vi "Controller.vi"() -> ()   [LabVIEW 2009]
uses:
  <vilib>/regexp/Match Regular Expression.xnode
  <vilib>/gmath/NI_Gmath.lvlib
  <vilib>/Analysis/NI_AALBase.lvlib
panel:
  out "Busy":bool
  in  "Tab Control":enum32{"Controls", "Calibrations", "Errors"}(tab)
  out "Standard Dev.":dbl caption="Std. Dev. (J)" format="%#_4e"
  out "Average":dbl caption="Mean (J)" format="%#_4e"
  in  "Averaging":string(combo)="10 s"
  in  "Tab Control 2":T1(tab)
  in  "Comments":string
  in  "Heads Numbers":i16[](array[numeric])
  in  "Heads":i32(listbox)
  in  "Pulsar Handle":i16
  out "Found?":bool
  out "Pulsar Info":string
  in  "OphirFastX":refnum<k7>(container)
  in  "Refreshing (ms)":i32=10
  in  "Window Time (us)":i32=1000
  in  "Ext. Trigger":bool=TRUE
  in  "Trigger Mode":string(combo)="Falling Edge"
  out "Check Lower Level":bool
  in  "Range (Numeric)":dbl[](array[numeric])
  in  "Max. Power (W)":dbl=12.0
  in  "Max. Energy (J)":dbl=1.2
  in  "Pulse Length":string(combo)
  in  "Wavelength (nm)":string(combo)
  in  "Range":string(combo)
  in  "Mode":string(combo)="Energy"
  in  "Autoscale":bool
  in  "Num 1":i32 min=0 max=9 step=1
  in  "Num 2":i32 min=-1 max=10 step=1
  in  "Num 3":i32 min=-1 max=10 step=1
  in  "Active Channels":T2={"A="=FALSE, "B="=FALSE, "C="=TRUE, "D="=TRUE}
  in  "Delays (s)":dbl[](array[numeric]) min=0.0 max=999.999999999999 format="%#_15f"
  in  "VISA Box":refnum<visa-resource-name>="GPIB0::15::INSTR"
  in  "Manual Mode":bool=TRUE
  in  "Modes":cluster{"A=":u16, "B=":u16, "C=":u16, "D=":u16} {"D=" items=["T0+", "A+", "B+", "C+"]; "C=" items=["T0+", "A+", "B+", "D+"]; "B=" items=["T0+", "A+", "C+", "D+"]; "A=" items=["T0+", "B+", "C+", "D+"]}
  in  "Num 4":i32 min=-1 max=10 step=1
  in  "Num 5":i32 min=-1 max=10 step=1
  in  "Num 6":i32 min=-1 max=10 step=1
  in  "Num 7":i32 min=-1 max=10 step=1
  in  "Num 8":i32 min=-1 max=10 step=1
  in  "Num 9":i32 min=-1 max=10 step=1
  in  "Num 10":i32 min=-1 max=10 step=1
  in  "Num 11":i32 min=-1 max=10 step=1
  in  "Num 12":i32 min=-1 max=10 step=1
  in  "Num 13":i32 min=-1 max=10 step=1
  in  "Num 14":i32 min=-1 max=10 step=1
  in  "Num 15":i32 min=-1 max=10 step=1
  in  "Channel":string(combo)="A"
  in  "Buffer Duration (s)":dbl=2.0
  in  "Add ConfigFile":bool=TRUE
  out "Sub-Buffer (# Points)":i32=5
  out "Error LED":bool
  out "Warning LED":bool
  out "OK LED":bool
  in  "Sub-buffer Sizes":u32[](array[numeric])
  in  "T0 (s)":u32[](array[numeric])
  in  "Simulate Values":bool
  in  "Buffer (units)":string(combo)="Minutes"
  in  "Buffer (size)":u32=5
  in  "Graph style":string(combo)="Chart"
  out "# OK":i32
  out "# Over Range":i32
  out "# Saturated":i32
  out "# Missing Pulses":i32
  out "# Points":i32
  in  "Min. Size (# Points)":i32=5
  in  "Export as .txt":bool
  out "Peak Power (W)":dbl
  out "Peak Energy (J)":dbl
  in  "Step Duration (s)":i32=10
  in  "# Steps":i32=20
  in  "Calibrate":bool
  in  "Rise":string(combo)="Synchronous"
  out "Display":dbl[][](graph)
  out "Measure":dbl caption="Energy (J)" format="%#_4e"
  in  "Slide Style":string(combo)="Absolute"
  in  "Slide (%,W,J)":dbl(slide) caption="Energy (J)" min=0.0 max=1.2 step=0.005 scale=0.0..1.2 scale format="%#_3f"
  in  "Acquire":bool=TRUE
  in  "Clear Graph":bool
  out "Abs Energies":dbl[](array[numeric])
  out "Calib Path":path=path "C:/Documents and Settings/loasis/My Documents/Guillaume/Powermeter/Godzilla Calibrations"
  in  "Titles":string[](array[string])=["Channel A", "Channel B", "Channel C", "Channel D", "Power (W)", "Energy (J)"]
  in  "RmvCalib":bool
  in  "Load list":bool
  in  "AddCalib":bool
  in  "List of calibrations":i32(listbox)=-1
  in  "Calibration":dbl[][](array[numeric])=[[0.000303, 0.000306, 0.000498714, 0.000498713, 0.05, 0.005], [0.000303, 0.000306, 0.000499714, 0.000499713, 0.1, 0.01], [0.000303, 0.000306, 0.000500314, 0.000500413, 0.2, 0.02], [0.000303, 0.000306, 0.000501314, 0.000501413, 0.5, 0.05], [0.000303, 0.000306, 0.000501914, 0.000501813, 1.0, 0.1], [0.000303, 0.000306, 0.000502414, 0.000502213, 2.0, 0.2], [0.000303, 0.000306, 0.000502514, 0.000502513, 3.0, 0.3], [0.000303, 0.000306, 0.000502714, 0.000502613, 4.0, 0.4], [0.000303, 0.000306, 0.000502914, 0.000502813, 5.0, 0.5], [0.000303, 0.000306, 0.000503014, 0.000503013, 6.1, 0.6], [0.000303, 0.000306, 0.000503114, 0.000503113, 7.0, 0.7], [0.000303, 0.000306, 0.000503214, 0.000503213, 8.0, 0.8], [0.000303, 0.000306, 0.000503314, 0.000503313, 9.0, 0.9], [0.000303, 0.000306, 0.000503314, 0.000503413, 9.7, 1.0]]
  out "Indexes":dbl[](array[numeric])
  out "Abs Powers":dbl[](array[numeric])
  in  "Tab Control 3":enum32{"Ophir", "Delay Box", "Saving/Loading"}(tab)
  out "Error Closing USB":errorcluster caption="error out"
  out "Error Getting Data":errorcluster caption="error out"
  out "Error Setting Head":errorcluster caption="error out"
  out "Error Initializing Head":errorcluster caption="error out"
  out "Error Reading Delay Box":errorcluster caption="error out"
  out "Error Writing Delay Box":errorcluster caption="error out"
  out "Error Exporting Text File":errorcluster caption="error out"
  out "Error Loading Dialog":errorcluster caption="error out"
  out "Error Deleting File":errorcluster caption="error out"
  out "Error Writing File":errorcluster caption="error out"
  out "Error Saving Dialog":errorcluster caption="error out"
  in  "Stop":bool
  # "LOASIS/LBNL - Power/Energy-meter Controller - Guillaume Plateau - Version 2.14 - May 2nd, 2010"
  # "(s)"
  # "(ms)"
  # "(us)"
  # "(ns)"
  # "(ps)"
  # "."
  # "Ophir Messages:"
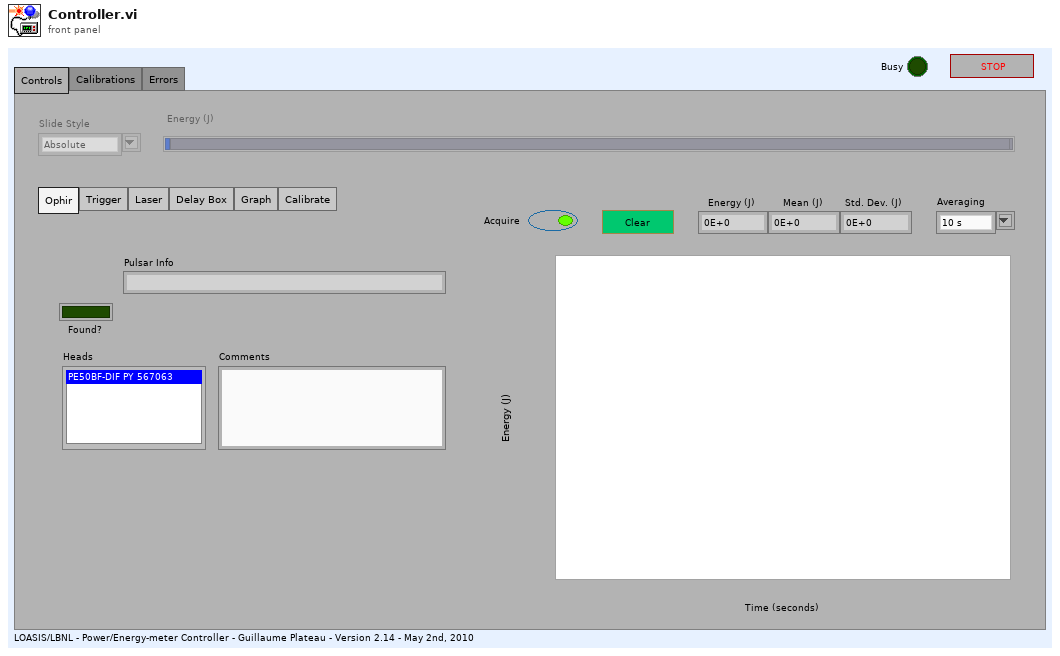
[diagram p1: front panel]
types:
  T1 = enum32{"Ophir", "Trigger", "Laser", "Delay Box", "Graph", "Calibrate"}
  T2 = cluster{"A=":bool, "B=":bool, "C=":bool, "D=":bool}
  T3 = cluster{"Ext. Trigger":bool, "Autoscale":bool, "Check Lower Level":bool, "VISA Box":refnum<visa-resource-name>, "Manual Mode":bool, "Delays (s)":dbl[], "Modes":cluster{"A=":u16, "B=":u16, "C=":u16, "D=":u16}, "Active Channels":cluster{"A=":bool, "B=":bool, "C=":bool, "D=":bool}, "Graph style":string, "Buffer (size)":u32, "Buffer (units)":string, "Min. Size (# Points)":i32, "Simulate Values":bool, "Calib Path":path, "Slide Style":string, "Max. Power (W)":dbl, "Max. Energy (J)":dbl, "Slide (%,W,J)":dbl, "Acquire":bool}
  T4 = cluster{"Ext. Trigger":bool, "Autoscale":bool, "Check Lower Level":bool, "VISA Box":refnum<visa-resource-name>, "Manual Mode":bool, "Delays (s)":dbl[], "Modes":cluster{"A=":u16, "B=":u16, "C=":u16, "D=":u16}, "Active Channels":cluster{"A=":bool, "B=":bool, "C=":bool, "D=":bool}, "Graph style":string, "Buffer (size)":u32, "Buffer (units)":string, "Min. Size (# Points)":i32, "Simulate Values":bool, "Calib Path":path, "Slide Style":string, "Max. Power (W)":dbl, "Max. Energy (J)":dbl, "Slide (%,W,J)":dbl, "Acquire":bool}[]
  T5 = cluster{"Graph (main buffer)":dbl[], "Times (main buffer)":u32[], "Graph (sub-buffer)":dbl[], "Times (sub-buffer)":u32[]}
  T6 = cluster{"Graph (main buffer)":dbl[], "Times (main buffer)":u32[], "Graph (sub-buffer)":dbl[], "Times (sub-buffer)":u32[]}[]
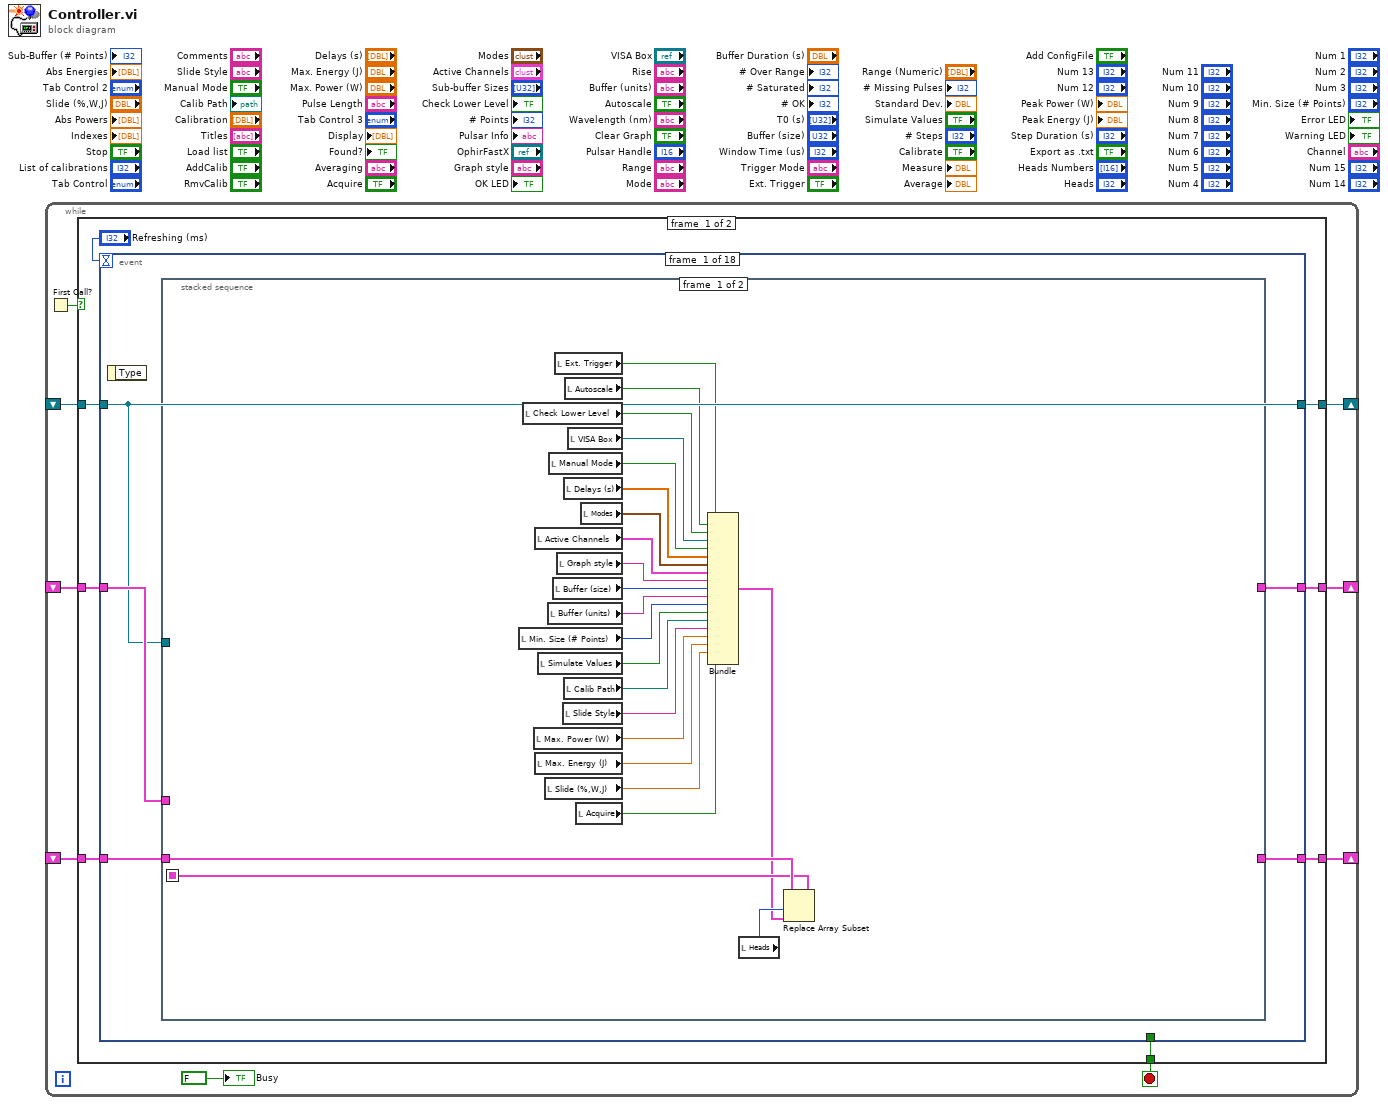
[diagram p0: block diagram]
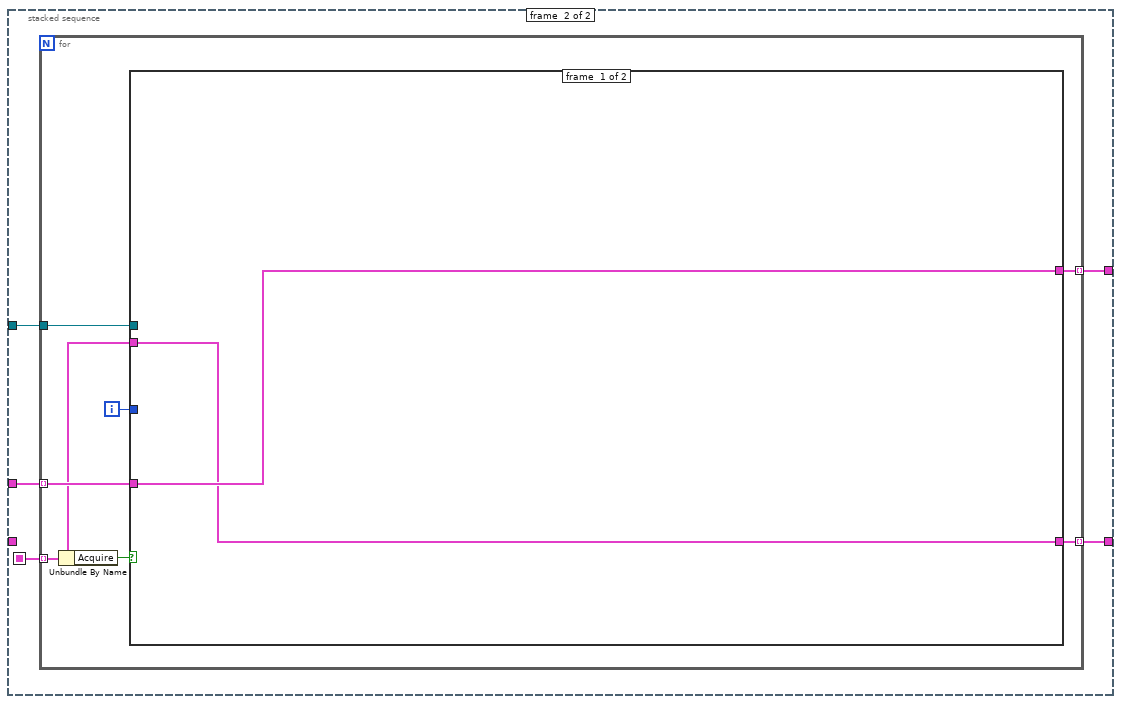
[diagram p2: hidden frame]
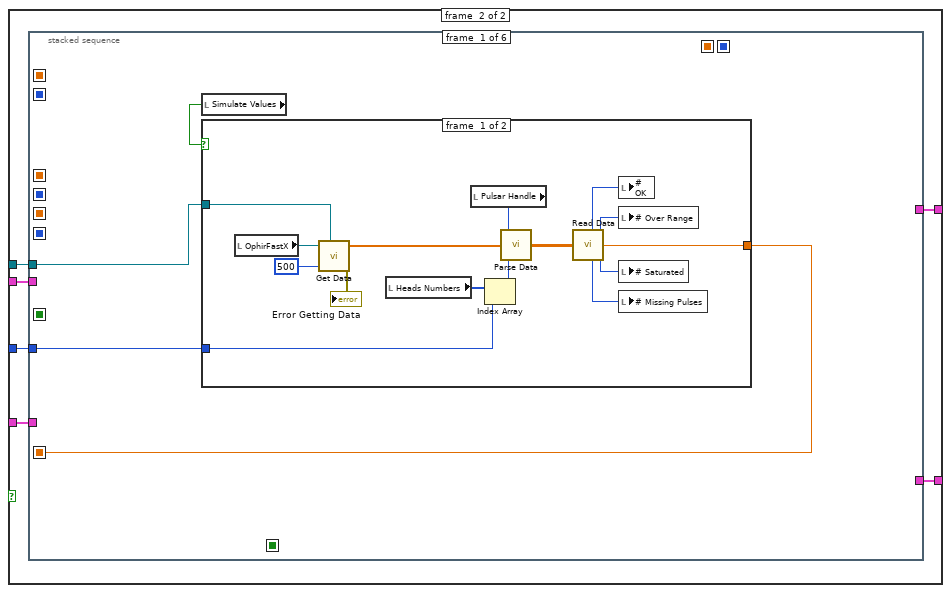
[diagram p3: hidden frame]
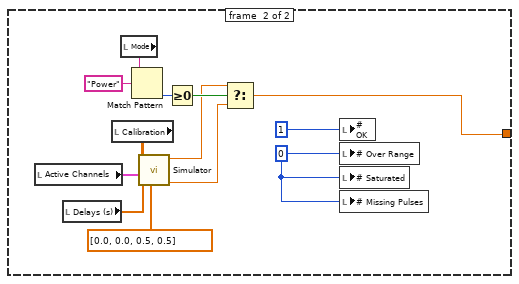
[diagram p4: hidden frame]
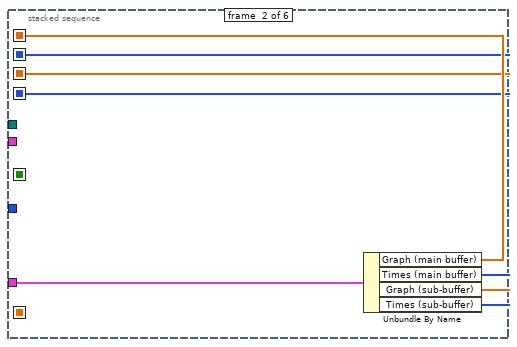
[diagram p5: hidden frame]
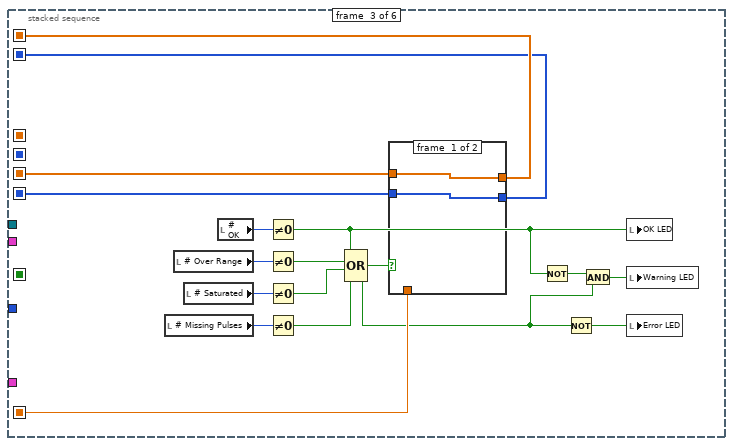
[diagram p6: hidden frame]
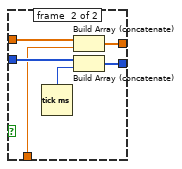
[diagram p7: hidden frame]
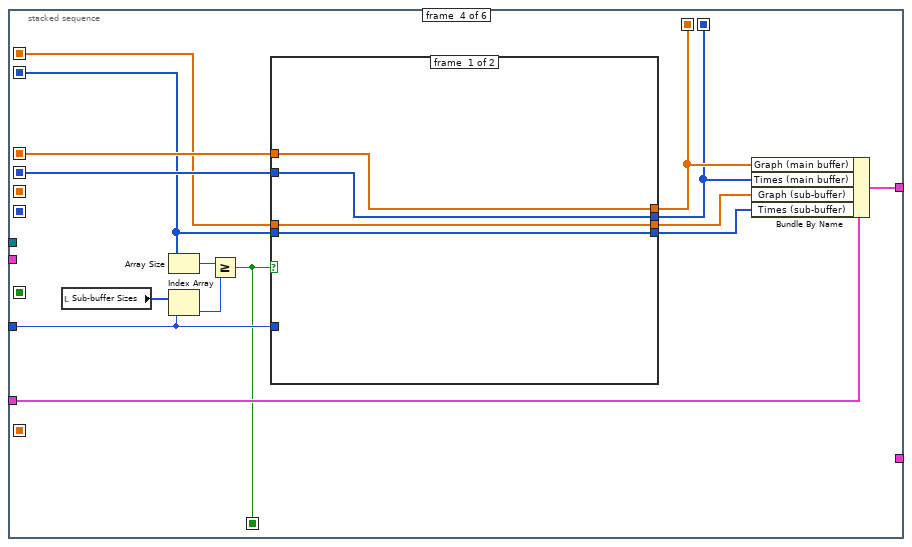
[diagram p8: hidden frame]
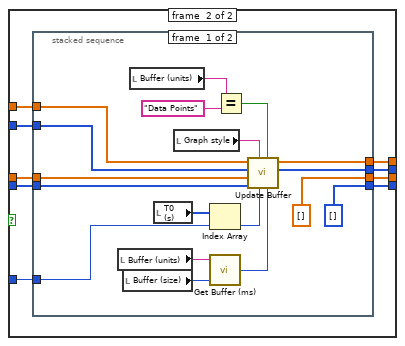
[diagram p9: hidden frame]
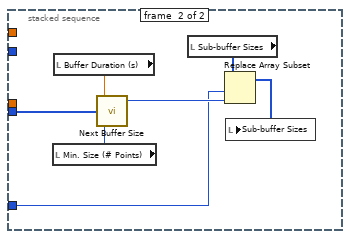
[diagram p10: hidden frame]
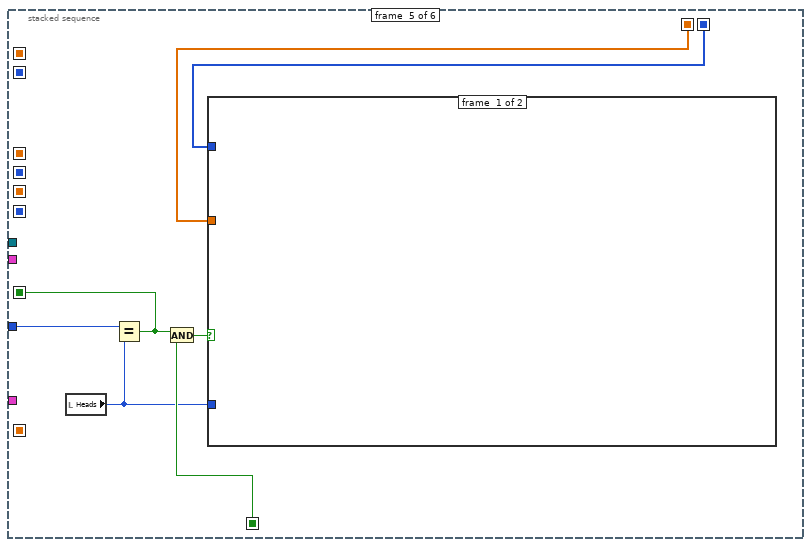
[diagram p11: hidden frame]
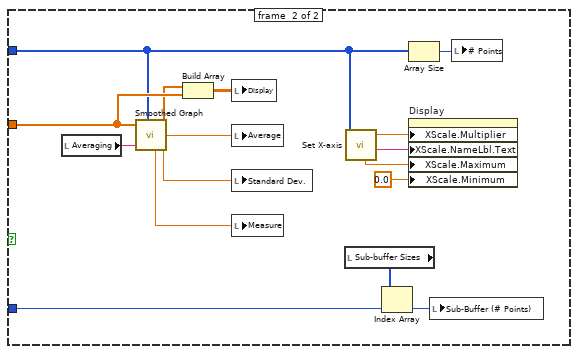
[diagram p12: hidden frame]
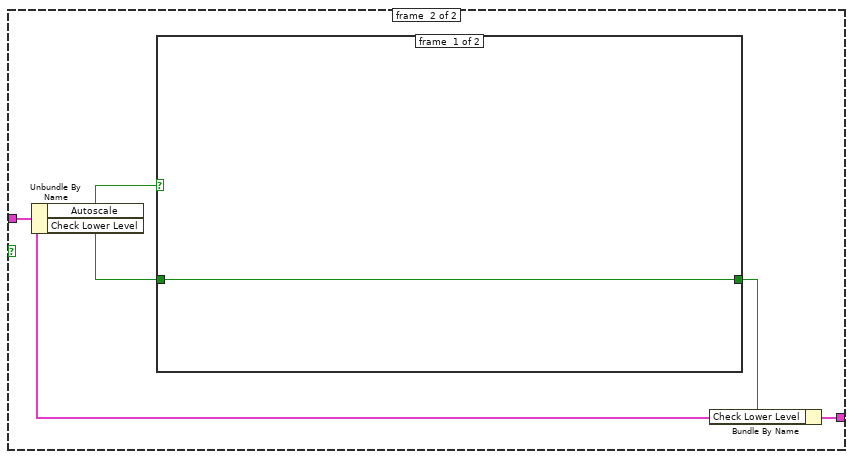
[diagram p14: hidden frame]
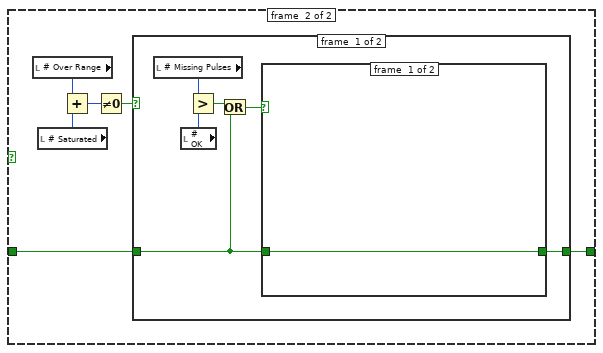
[diagram p15: hidden frame]
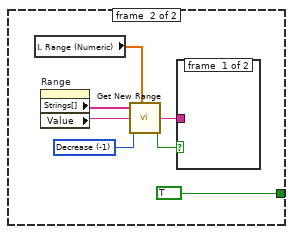
[diagram p16: hidden frame]
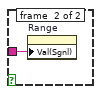
[diagram p17: hidden frame]
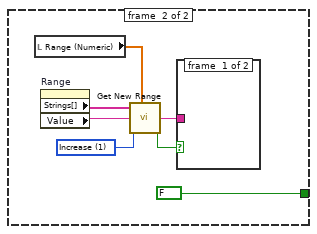
[diagram p18: hidden frame]
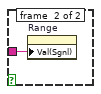
[diagram p19: hidden frame]
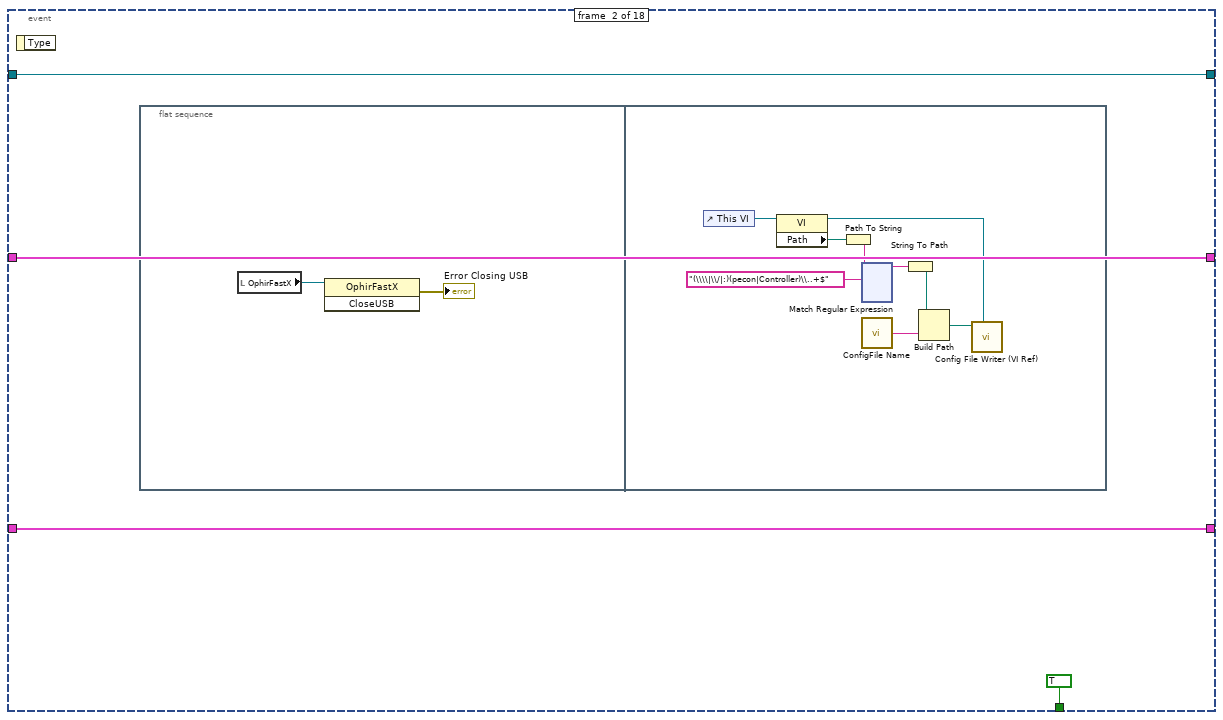
[diagram p20: hidden frame]
diagram:
  n1 = while {
    shift-right: [w7] -> _
    shift-left: _ -> [w6]
    shift-right: [w2] -> _
    shift-left: _ -> [w4]
    shift-right: [w1] -> _
    shift-left: _ -> [w3]
    stop <- w8 stop-if-true
    n2 = First Call?() -> (First Call?: T/F=w5:bool)
    n3 = case shown="False" w5 {
      tunnel: [w17 FALSE ("stop")] -> w8
      tunnel: [w11 w2302] -> w7
      tunnel: w6 -> [w12 _]
      tunnel: w3 -> [w13 w2299]
      tunnel: w4 -> [w15 _]
      tunnel: [w14 w2301] -> w2
      tunnel: [w10 w2300] -> w1
      frame #0 {
        n4 = event shown="[1] \"Stop\": Mouse Up" {
          selector: _ -> [_ _ _ _ _ _ _ _ _ _ _ _ _ _ _ _ _ _]
          dyn-events: _ -> [_ _ _ _ _ _ _ _ _ _ _ _ _ _ _ _ _ _]
          timeout: "Refreshing (ms)" -> [_ _ _ _ _ _ _ _ _ _ _ _ _ _ _ _ _ _]
          tunnel: [_ TRUE ("stop") _ _ _ _ _ _ _ _ _ _ _ _ _ _ _ _] -> w17
          tunnel: w15 -> [w21 w245 w366 w410 w424 w1004 w1060 w1112 w1149 w1291 w1351 w1403 w1791 w1818 w1847 w1884 w2220 w2286]
          tunnel: [w19 w245 w366 w409 w424 w1004 w1060 w1112 w1149 w1291 w1351 w1403 w1791 w1818 w1847 w1884 w2220 w2286] -> w14
          tunnel: w13 -> [w22 w243 w367 w407 w422 w1002 w1058 w1110 w1147 w1289 w1349 w1401 w1789 w1816 w1845 w1883 w2218 w2284]
          tunnel: w12 -> [w20 w244 w368 w408 w423 w1003 w1059 w1111 w1148 w1290 w1350 w1402 w1790 w1817 w1846 w1885 w2219 w2285]
          tunnel: [w20 w244 w368 w408 w423 w1003 w1059 w1111 w1148 w1290 w1350 w1402 w1790 w1817 w1846 w1885 w2219 w2285] -> w11
          tunnel: [w18 w243 w367 w407 w422 w1002 w1058 w1110 w1147 w1289 w1349 w1401 w1789 w1816 w1845 w1883 w2218 w2284] -> w10
          event #0 {
            n5 = event-data() -> ()  [unwired: 1 in, 1 out]
            n6 = stacked-sequence {
              seq-local: [w43 _] -> [_ w47]
              tunnel: w22 -> [w44 _]
              tunnel: [_ w50] -> w18
              tunnel: w20 -> [_ w49]
              tunnel: w21 -> [_ w48]
              tunnel: [_ w46] -> w19
              frame #0 {
                n7 = local read "Min. Size (# Points)"() -> (w24:i32)
                n8 = local read "Check Lower Level"() -> (w30:bool)
                n9 = local read "Max. Power (W)"() -> (w28:dbl)
                n10 = local read "Active Channels"() -> (w29:T2)
                n11 = local read "Max. Energy (J)"() -> (w27:dbl)
                n12 = local read "Simulate Values"() -> (w34:bool)
                n13 = local read "Slide (%,W,J)"() -> (w26:dbl)
                n14 = local read "Buffer (units)"() -> (w33:string)
                n15 = local read "Manual Mode"() -> (w39:bool)
                n16 = local read "Buffer (size)"() -> (w32:u32)
                n17 = local read "Ext. Trigger"() -> (w42:bool)
                n18 = local read "Graph style"() -> (w25:string)
                n19 = local read "Slide Style"() -> (w36:string)
                n20 = local read "Delays (s)"() -> (w38:dbl[])
                n21 = local read "Calib Path"() -> (w35:path)
                n22 = local read "Autoscale"() -> (w41:bool)
                n23 = local read "VISA Box"() -> (w40:refnum<visa-resource-name>)
                n24 = local read "Acquire"() -> (w37:bool)
                n25 = local read "Modes"() -> (w31:cluster{"A=":u16, "B=":u16, "C=":u16, "D=":u16})
                n26 = Bundle("Ext. Trigger"=w42, "Autoscale"=w41, "Check Lower Level"=w30, "VISA Box"=w40, "Manual Mode"=w39, "Delays (s)"=w38, "Modes"=w31, "Active Channels"=w29, "Graph style"=w25, "Buffer (size)"=w32, "Buffer (units)"=w33, "Min. Size (# Points)"=w24, "Simulate Values"=w34, "Calib Path"=w35, "Slide Style"=w36, "Max. Power (W)"=w28, "Max. Energy (J)"=w27, "Slide (%,W,J)"=w26, "Acquire"=w37) -> (w23:T3)  [unwired: 1 in]
                n27 = local read "Heads"() -> (w45:i32)
                n28 = Replace Array Subset(array=w44, new element=w23, index=w45) -> (w43:T4)
              }
              frame #1 {
                n29 = for {
                  tunnel: w49 -> [w57]
                  tunnel: w48 -> [w56] mode=indexing
                  tunnel: [w55] -> w46 mode=indexing
                  tunnel: w47 -> [w52] mode=indexing
                  tunnel: [w51] -> w50 mode=indexing
                  i -> [w54]
                  n30 = Unbundle By Name(w52) -> ("Acquire"=w53:bool)
                  n31 = case shown="True" w53 {
                    tunnel: w57 -> [_ w65]
                    tunnel: w56 -> [w59 w64]
                    tunnel: [w59 w63] -> w55
                    tunnel: w54 -> [_ w62]
                    tunnel: w52 -> [w58 w61]
                    tunnel: [w58 w60] -> w51
                    frame #0 {
                    }
                    frame #1 {
                      n32 = stacked-sequence {
                        seq-local: [_ w101 _ _ _ _] -> [_ _ _ w138 _ _]
                        seq-local: [_ w100 _ _ _ _] -> [_ _ _ w137 _ _]
                        seq-local: [_ w99 _ _ _ _] -> [_ _ w112 _ _ _]
                        seq-local: [_ w98 _ _ _ _] -> [_ _ w111 _ _ _]
                        seq-local: [_ _ w109 _ _ _] -> [_ _ _ w135 _ _]
                        seq-local: [_ _ w108 _ _ _] -> [_ _ _ w136 _ _]
                        seq-local: [_ _ _ w129 _ _] -> [_ _ _ _ w187 _]
                        seq-local: [_ _ _ w130 _ _] -> [_ _ _ _ w186 _]
                        seq-local: [_ _ _ w128 _ _] -> [_ _ _ _ w184 _]
                        seq-local: [w66 _ _ _ _ _] -> [_ _ w110 _ _ _]
                        seq-local: [_ _ _ _ w182 _] -> [_ _ _ _ _ w205]
                        tunnel: w65 -> [w69 _ _ _ _ _]
                        tunnel: w64 -> [_ w102 _ w134 _ _]
                        tunnel: w62 -> [w68 _ _ w139 w185 _]
                        tunnel: [_ _ _ w131 _ _] -> w63
                        tunnel: w61 -> [_ _ _ _ _ w206]
                        tunnel: [_ _ _ _ _ w204] -> w60
                        frame #0 {
                          n33 = local read "Simulate Values"() -> (w67:bool)
                          n34 = case shown="False" w67 {
                            tunnel: [w75 w86] -> w66
                            tunnel: w69 -> [w71 _]
                            tunnel: w68 -> [w70 _]
                            frame #0 {
                              n35 = local read "OphirFastX"() -> (w72:refnum<k7>)
                              n36 = call "Get Data.vi"("OphirFastX"=w72, "Notifier"=w71, "Timeout (ms)"=500 ("timeout in ms (-1)")) -> ("Data"=w81:dbl[], "Error"=→"Error Getting Data":errorcluster)  [unwired: 5 in]
                              n37 = local read "Heads Numbers"() -> (w74:i16[])
                              n38 = local read "Pulsar Handle"() -> (w82:i16)
                              n39 = Index Array(array=w74, index=w70) -> (element=w73:i16)
                              n40 = call "Parse Data.vi"("Head Channel"=w73, "Raw Data"=w81, "Pulsar Handle"=w82) -> ("Selected data"=w80:dbl[][])  [unwired: 2 in]
                              n41 = call "Read Data.vi"("Selected data"=w80) -> ("# OK"=w77:i32, "# Over Range"=w79:i32, "Data Point"=w75:dbl, "# Missing Pulses"=w76:i32, "# Saturated"=w78:i32)  [unwired: 4 in]
                              n42 = local write "# OK"(w77) -> ()
                              n43 = local write "# Over Range"(w79) -> ()
                              n44 = local write "# Saturated"(w78) -> ()
                              n45 = local write "# Missing Pulses"(w76) -> ()
                            }
                            frame #1 {
                              w87 = 0 ("# Over Range")
                              n46 = local read "Active Channels"() -> (w85:T2)
                              n47 = local read "Delays (s)"() -> (w96:dbl[])
                              n48 = local read "Calibration"() -> (w97:dbl[][])
                              n49 = local read "Mode"() -> (w94:string)
                              n50 = Match Pattern(string=w94, regular expression="Power") -> (offset past match=w92:i32)  [unwired: 1 in, 3 out]
                              n51 = call "Simulator.vi"("Proportions"=dbl[] [0.0, 0.0, 0.5, 0.5], "Delays (s)"=w96, "Active Channels"=w85, "Calibration"=w97) -> ("Output Energy (J)"=w89:dbl, "Output Power (W)"=w90:dbl)  [unwired: 6 in]
                              n52 = Greater Or Equal To 0?(x=w92) -> (x >= 0?=w91:bool)
                              n53 = Select(t=w90, s=w91, f=w89) -> (s? t:f=w86:dbl)
                              n54 = local write "# OK"(1 ("# OK")) -> ()
                              n55 = local write "# Over Range"(w87) -> ()
                              n56 = local write "# Saturated"(w87) -> ()
                              n57 = local write "# Missing Pulses"(w87) -> ()
                            }
                          }
                        }
                        frame #1 {
                          n58 = Unbundle By Name(w102) -> ("Graph (main buffer)"=w101:dbl[], "Times (main buffer)"=w100:u32[], "Graph (sub-buffer)"=w99:dbl[], "Times (sub-buffer)"=w98:u32[])
                        }
                        frame #2 {
                          n59 = local read "# Missing Pulses"() -> (w116:i32)
                          n60 = local read "# Over Range"() -> (w118:i32)
                          n61 = local read "# Saturated"() -> (w117:i32)
                          n62 = local read "# OK"() -> (w119:i32)
                          n63 = Not Equal To 0?(x=w119) -> (x != 0?=w106:bool)
                          n64 = Not Equal To 0?(x=w118) -> (x != 0?=w114:bool)
                          n65 = Not Equal To 0?(x=w117) -> (x != 0?=w113:bool)
                          n66 = Not Equal To 0?(x=w116) -> (x != 0?=w115:bool)
                          n67 = Compound Arithmetic op=OR(w106, w114, w113, w115) -> (w104:bool)
                          n68 = case shown="True" w104 {
                            tunnel: w112 -> [w121 w126]
                            tunnel: w111 -> [w120 w125]
                            tunnel: w110 -> [_ w124]
                            tunnel: [w121 w123] -> w109
                            tunnel: [w120 w122] -> w108
                            frame #0 {
                            }
                            frame #1 {
                              n69 = Tick Count (ms)() -> (millisecond timer value=w127:u32)
                              n70 = Build Array (concatenate)(w126, w124) -> (w123:dbl[])
                              n71 = Build Array (concatenate)(w125, w127) -> (w122:u32[])
                            }
                          }
                          n72 = Not(x=w106) -> (.not. x?=w105:bool)
                          n73 = Not(x=w104) -> (.not. x?=w107:bool)
                          n74 = And(x=w105, y=w104) -> (x .and. y?=w103:bool)
                          n75 = local write "OK LED"(w106) -> ()
                          n76 = local write "Warning LED"(w103) -> ()
                          n77 = local write "Error LED"(w107) -> ()
                        }
                        frame #3 {
                          n78 = local read "Sub-buffer Sizes"() -> (w141:u32[])
                          n79 = Array Size(array=w136) -> (size(s)=w142:i32)
                          n80 = Index Array(array=w141, index=w139) -> (element=w140:u32)
                          n81 = Greater Or Equal?(x=w142, y=w140) -> (x >= y?=w128:bool)
                          n82 = case shown="True" w128 {
                            tunnel: w139 -> [_ w155]
                            tunnel: w138 -> [w144 w150]
                            tunnel: w137 -> [w143 w149]
                            tunnel: w136 -> [w145 w154]
                            tunnel: w135 -> [w146 w153]
                            tunnel: [w144 w152] -> w130
                            tunnel: [w143 w151] -> w129
                            tunnel: [w146 w148] -> w133
                            tunnel: [w145 w147] -> w132
                            frame #0 {
                            }
                            frame #1 {
                              n83 = stacked-sequence {
                                tunnel: w155 -> [w165 w177]
                                tunnel: w154 -> [w163 w178]
                                tunnel: w153 -> [w162 _]
                                tunnel: [w161 _] -> w152
                                tunnel: [w160 _] -> w151
                                tunnel: w150 -> [w159 _]
                                tunnel: w149 -> [w158 _]
                                tunnel: [dbl[] [] ("Graph (out)") _] -> w148
                                tunnel: [u32[] [] ("Times (out)") _] -> w147
                                frame #0 {
                                n84 = local read "Buffer (units)"() -> (w173:string)
                                n85 = local read "Buffer (size)"() -> (w172:u32)
                                n86 = local read "Buffer (units)"() -> (w169:string)
                                n87 = local read "T0 (s)"() -> (w166:u32[])
                                n88 = local read "Graph style"() -> (w170:string)
                                n89 = Index Array(array=w166, index=w165) -> (element=w164:u32)
                                n90 = call "Get Buffer (ms).vi"("Buffer (size)"=w172, "Buffer (units)"=w173) -> ("Buffer (ms)"=w171:u32)  [unwired: 3 in]
                                n91 = Equal?(x=w169, y="Data Points") -> (x = y?=w167:bool)
                                n92 = call "Update Buffer.vi"("Buffer (ms)"=w171, "Data Points mode"=w167, "T0 (s)"=w164, "Graph style"=w170, "Times to add"=w163, "Values to add"=w162, "Times (in)"=w158, "Graph (in)"=w159) -> ("Times (out)"=w160:u32[], "Graph (out)"=w161:dbl[])  [unwired: 2 in]
                                }
                                frame #1 {
                                n93 = local read "Min. Size (# Points)"() -> (w176:i32)
                                n94 = local read "Buffer Duration (s)"() -> (w174:dbl)
                                n95 = call "Next Buffer Size.vi"("Min Size"=w176, "Times"=w178, "Buffer Duration (s)"=w174) -> ("Next buffer size"=w179:i32)  [unwired: 1 in, 1 out]
                                n96 = local read "Sub-buffer Sizes"() -> (w180:u32[])
                                n97 = Replace Array Subset(array=w180, new element=w179, index=w177) -> (w175:u32[])
                                n98 = local write "Sub-buffer Sizes"(w175) -> ()
                                }
                              }
                            }
                          }
                          n99 = Bundle By Name(cluster=w134, "Graph (main buffer)"=w130, "Times (main buffer)"=w129, "Graph (sub-buffer)"=w133, "Times (sub-buffer)"=w132) -> (w131:T5)
                        }
                        frame #4 {
                          n100 = local read "Heads"() -> (w181:i32)
                          n101 = Equal?(x=w185, y=w181) -> (x = y?=w182:bool)
                          n102 = And(x=w182, y=w184) -> (x .and. y?=w183:bool)
                          n103 = case shown="True" w183 {
                            tunnel: w186 -> [_ w201]
                            tunnel: w187 -> [_ w195]
                            tunnel: w181 -> [_ w188]
                            frame #0 {
                            }
                            frame #1 {
                              n104 = local read "Averaging"() -> (w202:string)
                              n105 = call "Smoothed Graph.vi"("Raw Graph"=w201, "Times"=w195, "Averaging"=w202) -> ("Avg Graph"=w200:dbl[], "Mean"=w198:dbl, "Last Value"=w197:dbl, "Std. Dev."=w196:dbl)  [unwired: 3 in]
                              n106 = Build Array(w200, w201) -> (w199:dbl[][])
                              n107 = local write "Display"(w199) -> ()
                              n108 = local write "Average"(w198) -> ()
                              n109 = local write "Standard Dev."(w196) -> ()
                              n110 = local write "Measure"(w197) -> ()
                              n111 = local read "Sub-buffer Sizes"() -> (w189:u32[])
                              n112 = call "Set X-axis.vi"("Times"=w195) -> ("X-label"=w193:string, "Multiplier"=w203:dbl, "X-Scale Maximum"=w192:dbl)  [unwired: 8 in]
                              n113 = Index Array(array=w189, index=w188) -> (element=w190:u32)
                              n114 = Array Size(array=w195) -> (size(s)=w194:i32)
                              n115 = property on="Display" class="WFGraph (strict)"("XScale.Multiplier"=w203, "XScale.NameLbl.Text"=w193, "XScale.Maximum"=w192, "XScale.Minimum"=0.0 ("X Scale.Range:Minimum")) -> ()  [unwired: 2 in, 2 out]
                              n116 = local write "Sub-Buffer (# Points)"(w190) -> ()
                              n117 = local write "# Points"(w194) -> ()
                            }
                          }
                        }
                        frame #5 {
                          n118 = case shown="True" w205 {
                            tunnel: w206 -> [w207 w208]
                            tunnel: [w207 w209] -> w204
                            frame #0 {
                            }
                            frame #1 {
                              n119 = Unbundle By Name(w208) -> ("Autoscale"=w212:bool, "Check Lower Level"=w211:bool)
                              n120 = case shown="True" w212 {
                                tunnel: w211 -> [w213 w215]
                                tunnel: [w213 w214] -> w210
                                frame #0 {
                                }
                                frame #1 {
                                n121 = local read "# Over Range"() -> (w219:i32)
                                n122 = local read "# Saturated"() -> (w218:i32)
                                n123 = Add(x=w219, y=w218) -> (x+y=w217:i32)
                                n124 = Not Equal To 0?(x=w217) -> (x != 0?=w216:bool)
                                n125 = case shown="False" w216 {
                                tunnel: w215 -> [w220 _]
                                tunnel: [w221 FALSE ("Check Lower Level")] -> w214
                                frame #0 {
                                n126 = local read "# Missing Pulses"() -> (w225:i32)
                                n127 = local read "# OK"() -> (w224:i32)
                                n128 = Greater?(x=w225, y=w224) -> (0:w223:bool)
                                n129 = Or(x=w223, y=w220) -> (x .or. y?=w222:bool)
                                n130 = case shown="True" w222 {
                                tunnel: [w226 TRUE ("Check Lower Level")] -> w221
                                tunnel: w220 -> [w226 _]
                                frame #0 {
                                }
                                frame #1 {
                                w231 = -1 items=["Decrease"=-1, "Increase"=1, "None"=0] ("Action")
                                n131 = local read "Range (Numeric)"() -> (w227:dbl[])
                                n132 = property on="Range" class="CmbBox"() -> ("Strings[]"=w233:string[], "Value"=w232:string)  [unwired: 2 in, 2 out]
                                n133 = call "Get New Range.vi"("Ranges"=w233, "Range (numeric)"=w227, "Range (char)"=w232, "Action"=w231) -> ("New Range"=w230:string, "New?"=w228:bool)  [unwired: 4 in]
                                n134 = case shown="True" w228 {
                                tunnel: w230 -> [_ w234]
                                frame #0 {
                                }
                                frame #1 {
                                n135 = property on="Range" class="CmbBox"("Val(Sgnl)"=w234) -> ()  [unwired: 2 in, 2 out]
                                }
                                }
                                }
                                }
                                }
                                frame #1 {
                                w239 = 1 items=["Decrease"=-1, "Increase"=1, "None"=0] ("Action")
                                n136 = local read "Range (Numeric)"() -> (w235:dbl[])
                                n137 = property on="Range" class="CmbBox"() -> ("Strings[]"=w241:string[], "Value"=w240:string)  [unwired: 2 in, 2 out]
                                n138 = call "Get New Range.vi"("Ranges"=w241, "Range (numeric)"=w235, "Range (char)"=w240, "Action"=w239) -> ("New Range"=w238:string, "New?"=w236:bool)  [unwired: 4 in]
                                n139 = case shown="True" w236 {
                                tunnel: w238 -> [_ w242]
                                frame #0 {
                                }
                                frame #1 {
                                n140 = property on="Range" class="CmbBox"("Val(Sgnl)"=w242) -> ()  [unwired: 2 in, 2 out]
                                }
                                }
                                }
                                }
                                }
                              }
                              n141 = Bundle By Name(cluster=w208, "Check Lower Level"=w210) -> (w209:T3)
                            }
                          }
                        }
                      }
                    }
                  }
                }
              }
            }
          }
          event #1 {
            n142 = event-data() -> ()  [unwired: 1 in, 1 out]
            n143 = flat-sequence {
              frame #0 {
                n144 = local read "OphirFastX"() -> (w248:refnum<k7>)
                n145 = invoke class="OphirFastX" method="CloseUSB"(reference=w248) -> (error out=→"Error Closing USB":errorcluster)  [unwired: 2 in, 2 out]
              }
              frame #1 {
                n146 = control-ref of="This VI"() -> (w257:refnum<vi>)
                n147 = property class="VI"(reference=w257) -> (reference out=w256:refnum<vi>, "Path"=w253:path)  [unwired: 1 in, 1 out]
                n148 = Path To String(path=w253) -> (string=w252:string)
                n149 = xnode "Match Regular Expression"("input string"=w252, "regular expression"="(\\\\|\\/|:)(pecon|Controller)\\..+$") -> ("before match"=w251:string)  [unwired: 4 in, 4 out]
                n150 = call "ConfigFile Name.vi"() -> ("ConfigFile Name"=w255:string)  [unwired: 5 in]
                n151 = String To Path(string=w251) -> (path=w250:path)
                n152 = Build Path(base path=w250, name or relative path=w255) -> (appended path=w249:path)
                n153 = call "Config File Writer (VI Ref).vi"("This VI"=w256, "Config File Path"=w249) -> ()  [unwired: 9 in, 1 out]
              }
            }
          }
          event #2 {
            n154 = event-data() -> ()  [unwired: 1 in, 1 out]
            n155 = flat-sequence {
              tunnel: w366 -> [w395]
              tunnel: [w373] -> w365
              tunnel: w365 -> [w396]
              frame #0 {
                w382 = "\t"
                n156 = local read "Heads"() -> (w393:i32)
                n157 = local read "Averaging"() -> (w369:string)
                n158 = Index Array(array=w395, index=w393) -> (element=w392:T5)
                n159 = property on="Display" class="WFGraph (strict)"() -> ("YScale.NameLbl.Text"=w371:string)  [unwired: 2 in, 2 out]
                n160 = Unbundle By Name(w392) -> ("Graph (main buffer)"=w380:dbl[], "Times (main buffer)"=w379:u32[])
                n161 = Concatenate Strings(w369, " Averaged " ("string"), w371) -> (w372:string)
                n162 = Array Size(array=w379) -> (size(s)=w391:i32)
                n163 = call "Set X-axis.vi"("Times"=w379) -> ("X-label"=w384:string, "Multiplier"=w390:dbl)  [unwired: 8 in, 1 out]
                n164 = Concatenate Strings(w384, w382, w371, w382, w372, "\r\n") -> (w377:string)
                n165 = local read "Averaging"() -> (w381:string)
                n166 = call <vilib>:"Ramp Pattern.vi"("samples"=w391) -> ("Ramp Pattern"=w389:dbl[])  [unwired: 9 in, 1 out]
                n167 = local write "Busy"(TRUE ("Busy")) -> ()
                n168 = Multiply(x=w390, y=w389) -> (x*y=w388:dbl[])
                n169 = call "Smoothed Graph.vi"("Raw Graph"=w380, "Times"=w379, "Averaging"=w381) -> ("Avg Graph"=w378:dbl[])  [unwired: 3 in, 3 out]
                n170 = Build Array(w388, w380, w378) -> (w387:dbl[][])
                n171 = Transpose 2D Array(2D array=w387) -> (transposed array=w385:dbl[][])
                n172 = Array To Spreadsheet String(array=w385, 3:"%3.12e" ("format string")) -> (spreadsheet string=w376:string)  [unwired: 1 in]
                n173 = Concatenate Strings(w377, w376) -> (w375:string)
                n174 = Write to Text File(text=w375) -> (refnum out=w373:refnum<file>, error out=→"Error Exporting Text File":errorcluster)  [unwired: 3 in, 1 out]
              }
              frame #1 {
                n175 = Not A Number/Path/Refnum?(number/path/refnum=w396) -> (NaN/Path/Refnum?=w400:bool)
                n176 = Not(x=w400) -> (.not. x?=w399:bool)
                n177 = local read "Add ConfigFile"() -> (w398:bool)
                n178 = Or(x=w398, y=w399) -> (x .or. y?=w397:bool)
                n179 = case shown="True" w397 {
                  tunnel: w396 -> [_ w401]
                  frame #0 {
                  }
                  frame #1 {
                    n180 = Close File(refnum=w401) -> (path=w403:path)  [unwired: 1 in, 1 out]
                    n181 = call "ConfigFile Name.vi"() -> ("ConfigFile Name"=w406:string)  [unwired: 5 in]
                    n182 = Strip Path(path=w403) -> (stripped path=w402:path)  [unwired: 1 out]
                    n183 = Build Path(base path=w402, name or relative path=w406) -> (appended path=w405:path)
                    n184 = control-ref of="This VI"() -> (w404:refnum<vi>)
                    n185 = call "Config File Writer (VI Ref).vi"("This VI"=w404, "Config File Path"=w405) -> ()  [unwired: 9 in, 1 out]
                  }
                }
              }
            }
          }
          event #3 {
            w420 = u32[] []  # Times (sub-buffer)
            w419 = dbl[] []  # Graph (sub-buffer)
            w418 = u32[] []  # Times (main buffer)
            w417 = dbl[] []  # Graph (main buffer)
            n186 = event-data() -> ()  [unwired: 1 in, 1 out]
            n187 = local write "Busy"(TRUE ("Busy")) -> ()
            n188 = Bundle("Graph (main buffer)"=w417, "Times (main buffer)"=w418, "Graph (sub-buffer)"=w419, "Times (sub-buffer)"=w420) -> (w416:T5)  [unwired: 1 in]
            n189 = local read "Heads"() -> (w421:i32)
            n190 = Replace Array Subset(array=w410, new element=w416, index=w421) -> (w409:T6)
            n191 = Tick Count (ms)() -> (millisecond timer value=w412:u32)
            n192 = local read "Heads"() -> (w414:i32)
            n193 = local read "T0 (s)"() -> (w413:u32[])
            n194 = Replace Array Subset(array=w413, new element=w412, index=w414) -> (w411:u32[])
            n195 = local write "T0 (s)"(w411) -> ()
          }
          event #4 {
            n196 = event-data() -> ()  [unwired: 1 in, 1 out]
            n197 = stacked-sequence {
              tunnel: w422 -> [w445 _ _ _ _ _ _ _ _]
              frame #0 {
                n198 = local write "Busy"(TRUE ("Busy")) -> ()
                n199 = local read "Heads"() -> (w447:i32)
                n200 = Index Array(array=w445, index=w447) -> (element=w425:T3)
                n201 = Unbundle(w425) -> ("Ext. Trigger"=w444:bool, "Autoscale"=w443:bool, "Check Lower Level"=w432:bool, "VISA Box"=w442:refnum<visa-resource-name>, "Manual Mode"=w441:bool, "Delays (s)"=w440:dbl[], "Modes"=w433:cluster{"A=":u16, "B=":u16, "C=":u16, "D=":u16}, "Active Channels"=w431:T2, "Graph style"=w427:string, "Buffer (size)"=w434:u32, "Buffer (units)"=w435:string, "Min. Size (# Points)"=w426:i32, "Simulate Values"=w436:bool, "Calib Path"=w437:path, "Slide Style"=w438:string, "Max. Power (W)"=w430:dbl, "Max. Energy (J)"=w429:dbl, "Slide (%,W,J)"=w428:dbl, "Acquire"=w439:bool)
                n202 = local write "Ext. Trigger"(w444) -> ()
                n203 = local write "Autoscale"(w443) -> ()
                n204 = local write "Check Lower Level"(w432) -> ()
                n205 = local write "VISA Box"(w442) -> ()
                n206 = local write "Manual Mode"(w441) -> ()
                n207 = local write "Delays (s)"(w440) -> ()
                n208 = local write "Modes"(w433) -> ()
                n209 = local write "Active Channels"(w431) -> ()
                n210 = local write "Graph style"(w427) -> ()
                n211 = local write "Buffer (size)"(w434) -> ()
                n212 = local write "Buffer (units)"(w435) -> ()
                n213 = local write "Min. Size (# Points)"(w426) -> ()
                n214 = local write "Simulate Values"(w436) -> ()
                n215 = local write "Calib Path"(w437) -> ()
                n216 = local write "Slide Style"(w438) -> ()
                n217 = local write "Max. Power (W)"(w430) -> ()
                n218 = local write "Max. Energy (J)"(w429) -> ()
                n219 = local write "Slide (%,W,J)"(w428) -> ()
                n220 = local write "Acquire"(w439) -> ()
              }
              frame #1 {
                n221 = local read "Acquire"() -> (w448:bool)
                n222 = case shown="False" w448 {
                  frame #0 {
                    n223 = local write "Display"(dbl[][] []) -> ()
                  }
                  frame #1 {
                  }
                }
              }
              frame #2 {
                n224 = local read "Manual Mode"() -> (w456:bool)
                n225 = local read "Autoscale"() -> (w452:bool)
                n226 = Select(t=u8 0, s=w456, f=u8 2) -> (s? t:f=w451:u8)
                n227 = Select(t=u8 2, s=w456, f=u8 0) -> (s? t:f=w450:u8)
                n228 = Select(t=u8 2, s=w452, f=u8 0) -> (s? t:f=w455:u8)
                n229 = property on="Range" class="CmbBox"("DisabledEnum"=w455) -> ()  [unwired: 2 in, 2 out]
                n230 = property on="VISA Box" class="VISAName"("DisabledEnum"=w451) -> ()  [unwired: 2 in, 2 out]
                n231 = property on="Delays (s)" class="Arr (strict)"("DisabledEnum"=w451) -> ()  [unwired: 2 in, 2 out]
                n232 = property on="Slide Style" class="CmbBox"("DisabledEnum"=w450) -> ()  [unwired: 2 in, 2 out]
                n233 = property on="Slide (%,W,J)" class="Slide (strict)"("DisabledEnum"=w450) -> ()  [unwired: 2 in, 2 out]
              }
              frame #3 {
                n234 = local read "Manual Mode"() -> (w462:bool)
                n235 = Select(t=u8 0, s=w462, f=u8 2) -> (s? t:f=w461:u8)
                n236 = property on="Num 4" class="DigNum (strict)"("DisabledEnum"=w461) -> ()  [unwired: 2 in, 2 out]
                n237 = property on="Num 5" class="DigNum (strict)"("DisabledEnum"=w461) -> ()  [unwired: 2 in, 2 out]
                n238 = property on="Num 6" class="DigNum (strict)"("DisabledEnum"=w461) -> ()  [unwired: 2 in, 2 out]
                n239 = property on="Num 7" class="DigNum (strict)"("DisabledEnum"=w461) -> ()  [unwired: 2 in, 2 out]
                n240 = property on="Num 8" class="DigNum (strict)"("DisabledEnum"=w461) -> ()  [unwired: 2 in, 2 out]
                n241 = property on="Num 9" class="DigNum (strict)"("DisabledEnum"=w461) -> ()  [unwired: 2 in, 2 out]
                n242 = property on="Num 10" class="DigNum (strict)"("DisabledEnum"=w461) -> ()  [unwired: 2 in, 2 out]
                n243 = property on="Num 11" class="DigNum (strict)"("DisabledEnum"=w461) -> ()  [unwired: 2 in, 2 out]
                n244 = property on="Num 12" class="DigNum (strict)"("DisabledEnum"=w461) -> ()  [unwired: 2 in, 2 out]
                n245 = property on="Num 13" class="DigNum (strict)"("DisabledEnum"=w461) -> ()  [unwired: 2 in, 2 out]
                n246 = property on="Num 14" class="DigNum (strict)"("DisabledEnum"=w461) -> ()  [unwired: 2 in, 2 out]
                n247 = property on="Num 15" class="DigNum (strict)"("DisabledEnum"=w461) -> ()  [unwired: 2 in, 2 out]
                n248 = property on="Channel" class="CmbBox"("DisabledEnum"=w461) -> ()  [unwired: 2 in, 2 out]
                n249 = property on="Num 1" class="DigNum (strict)"("DisabledEnum"=w461) -> ()  [unwired: 2 in, 2 out]
                n250 = property on="Num 2" class="DigNum (strict)"("DisabledEnum"=w461) -> ()  [unwired: 2 in, 2 out]
                n251 = property on="Num 3" class="DigNum (strict)"("DisabledEnum"=w461) -> ()  [unwired: 2 in, 2 out]
              }
              frame #4 {
                n252 = local read "Error Initializing Head"() -> (w474:errorcluster)
                n253 = local read "Heads Numbers"() -> (w472:i16[])
                n254 = property on="Heads" class="LstBox (strict)"() -> ("Item Names"=w473:string[], "Value"=w471:i32)  [unwired: 2 in, 2 out]
                n255 = local read "OphirFastX"() -> (w469:refnum<k7>)
                n256 = Index Array(array=w472, index=w471) -> (element=w466:i16)
                n257 = Index Array(array=w473, index=w471) -> (element=w470:string)
                n258 = local read "Pulsar Handle"() -> (w465:i16)
                n259 = control-ref of="Mode"() -> (w475:refnum<vi>)
                n260 = local read "Found?"() -> (w476:bool)
                n261 = call "Get Mode.vi"("Ref Mode"=w475, "Device Found?"=w476, "Head Info"=w470, "error in"=w474, "Head Channel"=w466, "Pulsar Handle"=w465, "OphirFastX (in)"=w469) -> ("error out"=w467:errorcluster, "OphirFastX (out)"=w468:refnum<k7>)  [unwired: 3 in]
                n262 = control-ref of="Range"() -> (w492:refnum<vi>)
                n263 = call "Get Range.vi"("Ref Range"=w492, "error in"=w467, "Head Channel"=w466, "Pulsar Handle"=w465, "OphirFastX (in)"=w468) -> ("error out"=w494:errorcluster, "OphirFastX (out)"=w493:refnum<k7>)  [unwired: 5 in]
                n264 = control-ref of="Wavelength (nm)"() -> (w491:refnum<vi>)
                n265 = call "Get Wavelength.vi"("Ref Wavelength"=w491, "error in"=w494, "Head Channel"=w466, "Pulsar Handle"=w465, "OphirFastX (in)"=w493) -> ("error out"=w489:errorcluster, "OphirFastX (out)"=w490:refnum<k7>)  [unwired: 5 in]
                n266 = control-ref of="Pulse Length"() -> (w488:refnum<vi>)
                n267 = call "Get Pulse Length.vi"("Ref Pulse Length"=w488, "error in"=w489, "Head Channel"=w466, "Pulsar Handle"=w465, "OphirFastX (in)"=w490) -> ("error out"=w486:errorcluster, "OphirFastX (out)"=w487:refnum<k7>)  [unwired: 5 in]
                n268 = control-ref of="Ext. Trigger"() -> (w477:refnum<vi>)
                n269 = call "Set Ext Trigger On-Off.vi"("Ext. Trigger"=w477, "error in"=w486, "Head Channel"=w466, "Pulsar Handle"=w465, "OphirFastX (in)"=w487) -> ("error out"=w484:errorcluster, "OphirFastX (out)"=w485:refnum<k7>)  [unwired: 5 in]
                n270 = control-ref of="Trigger Mode"() -> (w483:refnum<vi>)
                n271 = call "Get Ext Trigger Mode.vi"("Ref Trigger Mode"=w483, "error in"=w484, "Pulsar Handle"=w465, "OphirFastX (in)"=w485) -> ("error out"=w482:errorcluster, "OphirFastX (out)"=w479:refnum<k7>)  [unwired: 6 in]
                n272 = control-ref of="Window Time (us)"() -> (w480:refnum<vi>)
                n273 = call "Set Window Time.vi"("Ref Window Time"=w480, "Pulsar Handle"=w465, "OphirFastX (in)"=w479) -> ("OphirFastX (out)"=w478:refnum<k7>)  [unwired: 7 in, 1 out]
                n274 = call "Save Settings.vi"("error in"=w482, "Head Channel"=w466, "Pulsar Handle"=w465, "OphirFastX (in)"=w478) -> ("error out"=w495:errorcluster, "OphirFastX (out)"=w481:refnum<k7>)  [unwired: 6 in]
                n275 = local write "OphirFastX"(w481) -> ()
                n276 = local write "Error Initializing Head"(w495) -> ()
              }
              frame #5 {
                n277 = property on="Range" class="CmbBox"() -> ("Strings[]"=w497:string[])  [unwired: 2 in, 2 out]
                n278 = for {
                  tunnel: w497 -> [w498] mode=indexing
                  tunnel: [w501] -> w496 mode=indexing
                  n279 = xnode "Match Regular Expression"("input string"=w498, "regular expression"="[0-9]{1,4}\\.?[0-9]{0,2}") -> ("whole match"=w508:string)  [unwired: 4 in, 4 out]
                  n280 = xnode "Match Regular Expression"("input string"=w498, "regular expression"="m(J|W)") -> ("offset past match"=w500:i32)  [unwired: 4 in, 4 out]
                  n281 = xnode "Match Regular Expression"("input string"=w498, "regular expression"="u(J|W)") -> ("offset past match"=w499:i32)  [unwired: 4 in, 4 out]
                  n282 = Scan Value(string=w508, format string="%f") -> (value=w502:dbl)  [unwired: 1 in, 1 out]
                  n283 = Greater Or Equal To 0?(x=w500) -> (x >= 0?=w504:bool)
                  n284 = Greater Or Equal To 0?(x=w499) -> (x >= 0?=w503:bool)
                  n285 = case shown="False" w504 {
                    tunnel: w503 -> [w726 _]
                    tunnel: w502 -> [w725 w732]
                    tunnel: [w724 w731] -> w501
                    frame #0 {
                      n286 = case shown="True" w726 {
                        tunnel: w725 -> [w727 w730]
                        tunnel: [w727 w728] -> w724
                        frame #0 {
                        }
                        frame #1 {
                          n287 = Multiply(x=1e-06, y=w730) -> (x*y=w728:dbl)
                        }
                      }
                    }
                    frame #1 {
                      n288 = Multiply(x=0.001, y=w732) -> (x*y=w731:dbl)
                    }
                  }
                }
                n289 = local write "Range (Numeric)"(w496) -> ()
              }
              frame #6 {
                n290 = local read "Trigger Mode"() -> (w847:string)
                n291 = Match Pattern(string=w847, regular expression="Edge") -> (offset past match=w849:i32)  [unwired: 1 in, 3 out]
                n292 = local read "Ext. Trigger"() -> (w842:bool)
                n293 = Greater Or Equal To 0?(x=w849) -> (x >= 0?=w841:bool)
                n294 = And(x=w842, y=w841) -> (x .and. y?=w843:bool)
                n295 = Select(t=u8 0, s=w842, f=u8 2) -> (s? t:f=w850:u8)
                n296 = Select(t=u8 0, s=w843, f=u8 2) -> (s? t:f=w844:u8)
                n297 = property on="Trigger Mode" class="CmbBox"("DisabledEnum"=w850) -> ()  [unwired: 2 in, 2 out]
                n298 = property on="Window Time (us)" class="DigNum (strict)"("DisabledEnum"=w844) -> ()  [unwired: 2 in, 2 out]
              }
              frame #7 {
                n299 = local read "Mode"() -> (w866:string)
                n300 = Match Pattern(string=w866, regular expression="Power") -> (offset past match=w864:i32)  [unwired: 1 in, 3 out]
                n301 = Greater Or Equal To 0?(x=w864) -> (x >= 0?=w858:bool)
                n302 = Select(t="Power (W)" ("Y Scale.Name Label.Text"), s=w858, f="Energy (J)" ("Y Scale.Name Label.Text")) -> (s? t:f=w861:string)
                n303 = Select(t=" (W)" ("Y Scale.Name Label.Text"), s=w858, f=" (J)" ("Y Scale.Name Label.Text")) -> (s? t:f=w855:string)
                n304 = property on="Display" class="WFGraph (strict)"("YScale.NameLbl.Text"=w861) -> ()  [unwired: 2 in, 2 out]
                n305 = property on="Measure" class="DigNum (strict)"("Caption.Text"=w861) -> ()  [unwired: 2 in, 2 out]
                n306 = Concatenate Strings("Mean" ("string"), w855) -> (w854:string)
                n307 = Concatenate Strings("Std. Dev." ("string"), w855) -> (w853:string)
                n308 = property on="Average" class="DigNum (strict)"("Caption.Text"=w854) -> ()  [unwired: 2 in, 2 out]
                n309 = property on="Standard Dev." class="DigNum (strict)"("Caption.Text"=w853) -> ()  [unwired: 2 in, 2 out]
              }
              frame #8 {
                n310 = local read "Calib Path"() -> (w872:path)
                n311 = List Folder(path=w872) -> (filenames=w871:string[], error out=w875:errorcluster)  [unwired: 3 in, 2 out]
                n312 = local write "Error Loading Dialog"(w875) -> ()
                n313 = for {
                  tunnel: w871 -> [w878] mode=indexing
                  shift-right: [w881] -> w868
                  shift-left: string[] [] -> [w882]
                  tunnel: ".*[0-9]{4}_[0-9]{4}.*\\.txt" ("pattern") -> [w880]
                  n314 = xnode "Match Regular Expression"("input string"=w878, "regular expression"=w880) -> ("offset past match"=w883:i32)  [unwired: 4 in, 4 out]
                  n315 = Less Than 0?(x=w883) -> (x < 0?=w877:bool)
                  n316 = Match Pattern(string=w878, regular expression="\\.txt") -> (before substring=w876:string)  [unwired: 1 in, 3 out]
                  n317 = case shown="False" w877 {
                    tunnel: w876 -> [w886 _]
                    tunnel: w882 -> [w885 w887]
                    tunnel: [w884 w887] -> w881
                    frame #0 {
                      n318 = Build Array (concatenate)(w885, w886) -> (w884:string[])
                    }
                    frame #1 {
                    }
                  }
                }
                n319 = Empty Array?(array=w868) -> (empty?=w874:bool)
                n320 = case shown="False" w874 {
                  tunnel: w868 -> [w997 _]
                  tunnel: [w995 -1 ("lower limit")] -> w873
                  frame #0 {
                    n321 = Array Size(array=w997) -> (size(s)=w998:i32)
                    n322 = local read "List of calibrations"() -> (w996:i32)
                    n323 = Decrement(x=w998) -> (x-1=w1000:i32)
                    n324 = In Range and Coerce(upper limit=w1000, x=w996, lower limit=0) -> (coerced(x)=w995:i32)  [unwired: 1 out]
                  }
                  frame #1 {
                  }
                }
                n325 = call "Sort name chrono.vi"("Names"=w868) -> ("Names Sorted"=w867:string[])  [unwired: 4 in]
                n326 = property on="List of calibrations" class="LstBox (strict)"("Item Names"=w867, "Val(Sgnl)"=w873) -> ()  [unwired: 2 in, 2 out]
              }
            }
          }
          event #5 {
            n327 = event-data() -> ()  [unwired: 1 in, 1 out]
            n328 = stacked-sequence {
              frame #0 {
                n329 = local read "List of calibrations"() -> (w1016:i32)
                n330 = Less Than 0?(x=w1016) -> (x < 0?=w1011:bool)
                n331 = local read "Manual Mode"() -> (w1010:bool)
                n332 = Select(t=TRUE, s=w1011, f=w1010) -> (s? t:f=w1008:bool)
                n333 = local read "Autoscale"() -> (w1017:bool)
                n334 = local write "Manual Mode"(w1008) -> ()
                n335 = case shown="False" w1008 {
                  frame #0 {
                    n336 = local read "Slide (%,W,J)"() -> (w1021:dbl)
                    n337 = property on="Slide (%,W,J)" class="Slide (strict)"("Val(Sgnl)"=w1021) -> ()  [unwired: 2 in, 2 out]
                  }
                  frame #1 {
                  }
                }
                n338 = Select(t=u8 2, s=w1017, f=u8 0) -> (s? t:f=w1020:u8)
                n339 = property on="Range" class="CmbBox"("DisabledEnum"=w1020) -> ()  [unwired: 2 in, 2 out]
                n340 = Select(t=u8 0, s=w1008, f=u8 2) -> (s? t:f=w1007:u8)
                n341 = Select(t=u8 2, s=w1008, f=u8 0) -> (s? t:f=w1006:u8)
                n342 = property on="VISA Box" class="VISAName"("DisabledEnum"=w1007) -> ()  [unwired: 2 in, 2 out]
                n343 = property on="Delays (s)" class="Arr (strict)"("DisabledEnum"=w1007) -> ()  [unwired: 2 in, 2 out]
                n344 = property on="Slide Style" class="CmbBox"("DisabledEnum"=w1006) -> ()  [unwired: 2 in, 2 out]
                n345 = property on="Slide (%,W,J)" class="Slide (strict)"("DisabledEnum"=w1006) -> ()  [unwired: 2 in, 2 out]
              }
              frame #1 {
                n346 = local read "Manual Mode"() -> (w1023:bool)
                n347 = Select(t=u8 0, s=w1023, f=u8 2) -> (s? t:f=w1022:u8)
                n348 = property on="Num 4" class="DigNum (strict)"("DisabledEnum"=w1022) -> ()  [unwired: 2 in, 2 out]
                n349 = property on="Num 5" class="DigNum (strict)"("DisabledEnum"=w1022) -> ()  [unwired: 2 in, 2 out]
                n350 = property on="Num 6" class="DigNum (strict)"("DisabledEnum"=w1022) -> ()  [unwired: 2 in, 2 out]
                n351 = property on="Num 7" class="DigNum (strict)"("DisabledEnum"=w1022) -> ()  [unwired: 2 in, 2 out]
                n352 = property on="Num 8" class="DigNum (strict)"("DisabledEnum"=w1022) -> ()  [unwired: 2 in, 2 out]
                n353 = property on="Num 9" class="DigNum (strict)"("DisabledEnum"=w1022) -> ()  [unwired: 2 in, 2 out]
                n354 = property on="Num 10" class="DigNum (strict)"("DisabledEnum"=w1022) -> ()  [unwired: 2 in, 2 out]
                n355 = property on="Num 11" class="DigNum (strict)"("DisabledEnum"=w1022) -> ()  [unwired: 2 in, 2 out]
                n356 = property on="Num 12" class="DigNum (strict)"("DisabledEnum"=w1022) -> ()  [unwired: 2 in, 2 out]
                n357 = property on="Num 13" class="DigNum (strict)"("DisabledEnum"=w1022) -> ()  [unwired: 2 in, 2 out]
                n358 = property on="Num 14" class="DigNum (strict)"("DisabledEnum"=w1022) -> ()  [unwired: 2 in, 2 out]
                n359 = property on="Num 15" class="DigNum (strict)"("DisabledEnum"=w1022) -> ()  [unwired: 2 in, 2 out]
                n360 = property on="Channel" class="CmbBox"("DisabledEnum"=w1022) -> ()  [unwired: 2 in, 2 out]
                n361 = property on="Num 1" class="DigNum (strict)"("DisabledEnum"=w1022) -> ()  [unwired: 2 in, 2 out]
                n362 = property on="Num 2" class="DigNum (strict)"("DisabledEnum"=w1022) -> ()  [unwired: 2 in, 2 out]
                n363 = property on="Num 3" class="DigNum (strict)"("DisabledEnum"=w1022) -> ()  [unwired: 2 in, 2 out]
              }
              frame #2 {
                w1027 = i16 15 ("width (-)")
                n364 = local read "Channel"() -> (w1033:string)
                n365 = case shown="\"A\", Default" w1033 {
                  tunnel: [0 1 2 3] -> w1032
                  frame #0 {
                  }
                  frame #1 {
                  }
                  frame #2 {
                  }
                  frame #3 {
                  }
                }
                n366 = local read "Delays (s)"() -> (w1031:dbl[])
                n367 = Index Array(array=w1031, index=w1032) -> (element=w1026:dbl)
                n368 = Multiply(x=1000000000000.0, y=w1026) -> (x*y=w1029:dbl)
                n369 = Number To Decimal String(number=w1029, width (-)=w1027) -> (decimal integer string=w1028:string)
                n370 = for {
                  N: w1027 -> [_]
                  tunnel: w1028 -> [w1038]
                  i -> [w1035]
                  n371 = String Subset(string=w1038, offset (0)=w1035, length (rest)=1 ("length (rest)")) -> (substring=w1036:string)
                  n372 = Decimal String To Number(string=w1036) -> (number=w1034:i32)  [unwired: 2 in, 1 out]
                  n373 = case shown="0, Default" w1035 {
                    tunnel: w1034 -> [w1039 w1040 w1041 w1042 w1043 w1044 w1045 w1046 w1047 w1048 w1049 w1050 w1051 w1052 w1053]
                    frame #0 {
                      n374 = local write "Num 1"(w1039) -> ()
                    }
                    frame #1 {
                      n375 = local write "Num 2"(w1040) -> ()
                    }
                    frame #2 {
                      n376 = local write "Num 3"(w1041) -> ()
                    }
                    frame #3 {
                      n377 = local write "Num 4"(w1042) -> ()
                    }
                    frame #4 {
                      n378 = local write "Num 5"(w1043) -> ()
                    }
                    frame #5 {
                      n379 = local write "Num 6"(w1044) -> ()
                    }
                    frame #6 {
                      n380 = local write "Num 7"(w1045) -> ()
                    }
                    frame #7 {
                      n381 = local write "Num 8"(w1046) -> ()
                    }
                    frame #8 {
                      n382 = local write "Num 9"(w1047) -> ()
                    }
                    frame #9 {
                      n383 = local write "Num 10"(w1048) -> ()
                    }
                    frame #10 {
                      n384 = local write "Num 11"(w1049) -> ()
                    }
                    frame #11 {
                      n385 = local write "Num 12"(w1050) -> ()
                    }
                    frame #12 {
                      n386 = local write "Num 13"(w1051) -> ()
                    }
                    frame #13 {
                      n387 = local write "Num 14"(w1052) -> ()
                    }
                    frame #14 {
                      n388 = local write "Num 15"(w1053) -> ()
                    }
                  }
                }
              }
            }
            n389 = local write "Busy"(TRUE ("Busy")) -> ()
          }
          event #6 {
            n390 = event-data() -> ()  [unwired: 1 in, 1 out]
            n391 = stacked-sequence {
              seq-local: [w1062 _] -> [_ w1098]
              frame #0 {
                n392 = control-ref of="List of calibrations"() -> (w1064:refnum<vi>)
                n393 = local write "Busy"(TRUE ("Busy")) -> ()
                n394 = call "Build Default Name.vi"("List of calibrations"=w1064) -> ("Default name"=w1063:string)  [unwired: 4 in]
                n395 = local read "Calib Path"() -> (w1070:path)
                n396 = call "File Dialog"("start path"=w1070, "prompt"="Save current calibration as:", "default name"=w1063, "pattern (all files)"="*.txt", "pattern label"="Text Files") -> ("selected path"=w1062:path, "cancelled"=w1066:bool, "error out"=→"Error Saving Dialog":errorcluster)  [unwired: 7 in, 1 out]
                n397 = case shown="False" w1066 {
                  tunnel: w1062 -> [w1079 _]
                  frame #0 {
                    n398 = local read "Titles"() -> (w1074:string[])
                    n399 = Index Array(array=w1074) -> (element=w1071:string)  [unwired: 1 in]
                    n400 = Array Subset(array=w1074, index=1) -> (w1072:string[])  [unwired: 1 in]
                    n401 = for {
                      tunnel: w1072 -> [w1086] mode=indexing
                      shift-right: [w1084] -> w1077
                      shift-left: w1071 -> [w1085]
                      n402 = Concatenate Strings(w1085, "\t", w1086) -> (w1084:string)
                    }
                    n403 = local read "Calibration"() -> (w1083:dbl[][])
                    n404 = Concatenate Strings(w1077, "\r") -> (w1075:string)
                    n405 = Array To Spreadsheet String(array=w1083, 3:"%3.12f" ("format string")) -> (spreadsheet string=w1081:string)  [unwired: 1 in]
                    n406 = Concatenate Strings(w1075, w1081) -> (w1080:string)
                    n407 = Write to Text File(file (use dialog)=w1079, text=w1080) -> (error out=→"Error Writing File":errorcluster)  [unwired: 2 in, 2 out]
                  }
                  frame #1 {
                  }
                }
              }
              frame #1 {
                # "1. Find \\name.\n2. Find name\n(so name can include dots)"
                n408 = Path To String(path=w1098) -> (string=w1097:string)
                n409 = Match Pattern(string=w1097, regular expression="\\\\[^\\\\]*\\.") -> (before substring=w1091:string, match substring=w1094:string)  [unwired: 1 in, 2 out]
                n410 = String To Path(string=w1091) -> (path=w1090:path)
                n411 = local read "Calib Path"() -> (w1089:path)
                n412 = property on="List of calibrations" class="LstBox (strict)"() -> ("Item Names"=w1093:string[])  [unwired: 2 in, 2 out]
                n413 = Equal?(x=w1089, y=w1090) -> (x = y?=w1088:bool)
                n414 = Match Pattern(string=w1094, regular expression="[^\\\\].*[^\\.]") -> (match substring=w1092:string)  [unwired: 1 in, 3 out]
                n415 = case shown="True" w1088 {
                  tunnel: w1093 -> [_ w1103]
                  tunnel: w1092 -> [_ w1099]
                  frame #0 {
                  }
                  frame #1 {
                    n416 = Match First String(2:w1103, 3:w1099) -> (0:w1105:i32)  [unwired: 1 out]
                    n417 = Less Than 0?(x=w1105) -> (x < 0?=w1104:bool)
                    n418 = case shown="True" w1104 {
                      tunnel: w1099 -> [_ w1108]
                      tunnel: w1103 -> [w1106 w1109]
                      tunnel: [w1106 w1107] -> w1102
                      frame #0 {
                      }
                      frame #1 {
                        n419 = Build Array (concatenate)(w1108, w1109) -> (w1107:string[])
                      }
                    }
                    n420 = call "Sort name chrono.vi"("Names"=w1102) -> ("Names Sorted"=w1101:string[])  [unwired: 4 in]
                    n421 = Match First String(2:w1101, 3:w1099) -> (0:w1100:i32)  [unwired: 1 out]
                    n422 = property on="List of calibrations" class="LstBox (strict)"("Item Names"=w1101, "Val(Sgnl)"=w1100) -> ()  [unwired: 2 in, 2 out]
                  }
                }
              }
            }
          }
          event #7 {
            n423 = event-data() -> ()  [unwired: 1 in, 1 out]
            n424 = stacked-sequence {
              frame #0 {
                n425 = property on="List of calibrations" class="LstBox (strict)"() -> ("Item Names"=w1120:string[], "Value"=w1116:i32)  [unwired: 2 in, 2 out]
                n426 = local write "Busy"(TRUE ("Busy")) -> ()
                n427 = Less Than 0?(x=w1116) -> (x < 0?=w1121:bool)
                n428 = case shown="False" w1121 {
                  tunnel: w1120 -> [w1127 w1146]
                  tunnel: w1116 -> [w1128 _]
                  tunnel: [w1125 w1146] -> w1119
                  frame #0 {
                    n429 = Index Array(array=w1127, index=w1128) -> (element=w1124:string)
                    n430 = Concatenate Strings(w1124, ".txt") -> (w1123:string)
                    n431 = local read "Calib Path"() -> (w1126:path)
                    n432 = Build Path(base path=w1126, name or relative path=w1123) -> (appended path=w1131:path)
                    n433 = call <vilib>:"Check if File or Folder Exists.vi"("path"=w1131) -> ("file or folder exists?"=w1130:bool, "dup path"=w1129:path)  [unwired: 8 in, 1 out]
                    n434 = case shown="True" w1130 {
                      tunnel: w1129 -> [_ w1140]
                      tunnel: w1128 -> [w1132 w1138]
                      tunnel: w1127 -> [w1133 w1137]
                      tunnel: w1123 -> [_ _]
                      tunnel: [w1134 w1136] -> w1125
                      frame #0 {
                        n435 = Delete From Array(array=w1133, index=w1132) -> (array with subset deleted=w1134:string[])  [unwired: 1 in, 1 out]
                      }
                      frame #1 {
                        n436 = Delete(path (use dialog)=w1140, confirm (F)=TRUE) -> (cancelled=w1139:bool, error out=→"Error Deleting File":errorcluster)  [unwired: 3 in, 1 out]
                        n437 = case shown="False" w1139 {
                          tunnel: w1138 -> [w1144 _]
                          tunnel: w1137 -> [w1143 w1145]
                          tunnel: [w1142 w1145] -> w1136
                          frame #0 {
                            n438 = Delete From Array(array=w1143, index=w1144) -> (array with subset deleted=w1142:string[])  [unwired: 1 in, 1 out]
                          }
                          frame #1 {
                          }
                        }
                      }
                    }
                  }
                  frame #1 {
                  }
                }
                n439 = Array Size(array=w1119) -> (size(s)=w1118:i32)
                n440 = Decrement(x=w1118) -> (x-1=w1114:i32)
                n441 = In Range and Coerce(upper limit=w1114, x=w1116, lower limit=0) -> (coerced(x)=w1115:i32)  [unwired: 1 out]
                n442 = property on="List of calibrations" class="LstBox (strict)"("Item Names"=w1119, "Val(Sgnl)"=w1115) -> ()  [unwired: 2 in, 2 out]
              }
            }
          }
          event #8 {
            n443 = event-data() -> ()  [unwired: 1 in, 1 out]
            n444 = stacked-sequence {
              frame #0 {
                n445 = local read "Calib Path"() -> (w1162:path)
                n446 = local write "Busy"(TRUE ("Busy")) -> ()
                n447 = call "File Dialog3"("start path"=w1162, "prompt"="Select calibration folder") -> ("selected path"=w1158:path, "error out"=w1152:errorcluster)  [unwired: 10 in, 2 out]
                n448 = local write "Calib Path"(w1158) -> ()
                n449 = List Folder(path=w1158, error in=w1152) -> (filenames=w1157:string[], error out=→"Error Loading Dialog":errorcluster)  [unwired: 2 in, 2 out]
                n450 = for {
                  tunnel: w1157 -> [w1165] mode=indexing
                  shift-right: [w1168] -> w1154
                  shift-left: string[] [] -> [w1169]
                  tunnel: ".*[0-9]{4}_[0-9]{4}.*\\.txt" ("pattern") -> [w1167]
                  n451 = xnode "Match Regular Expression"("input string"=w1165, "regular expression"=w1167) -> ("offset past match"=w1170:i32)  [unwired: 4 in, 4 out]
                  n452 = Less Than 0?(x=w1170) -> (x < 0?=w1164:bool)
                  n453 = Match Pattern(string=w1165, regular expression="\\.txt") -> (before substring=w1163:string)  [unwired: 1 in, 3 out]
                  n454 = case shown="False" w1164 {
                    tunnel: w1163 -> [w1173 _]
                    tunnel: w1169 -> [w1172 w1174]
                    tunnel: [w1171 w1174] -> w1168
                    frame #0 {
                      n455 = Build Array (concatenate)(w1172, w1173) -> (w1171:string[])
                    }
                    frame #1 {
                    }
                  }
                }
                n456 = Empty Array?(array=w1154) -> (empty?=w1160:bool)
                n457 = case shown="False" w1160 {
                  tunnel: w1154 -> [w1284 _]
                  tunnel: [w1282 -1 ("lower limit")] -> w1159
                  frame #0 {
                    n458 = Array Size(array=w1284) -> (size(s)=w1285:i32)
                    n459 = local read "List of calibrations"() -> (w1283:i32)
                    n460 = Decrement(x=w1285) -> (x-1=w1287:i32)
                    n461 = In Range and Coerce(upper limit=w1287, x=w1283, lower limit=0) -> (coerced(x)=w1282:i32)  [unwired: 1 out]
                  }
                  frame #1 {
                  }
                }
                n462 = call "Sort name chrono.vi"("Names"=w1154) -> ("Names Sorted"=w1153:string[])  [unwired: 4 in]
                n463 = property on="List of calibrations" class="LstBox (strict)"("Item Names"=w1153, "Val(Sgnl)"=w1159) -> ()  [unwired: 2 in, 2 out]
              }
            }
          }
          event #9 {
            n464 = event-data() -> ()  [unwired: 1 in, 1 out]
            n465 = stacked-sequence {
              frame #0 {
                n466 = property on="List of calibrations" class="LstBox (strict)"() -> ("Item Names"=w1294:string[], "Value"=w1293:i32)  [unwired: 2 in, 2 out]
                n467 = local write "Busy"(TRUE ("Busy")) -> ()
                n468 = Empty Array?(array=w1294) -> (empty?=w1295:bool)
                n469 = case shown="True" w1295 {
                  tunnel: w1294 -> [w1296 _]
                  tunnel: w1293 -> [w1305 _]
                  tunnel: w1293 -> [w1297 _]
                  frame #0 {
                    n470 = Index Array(array=w1296, index=w1305) -> (element=w1300:string)
                    n471 = Concatenate Strings(w1300, ".txt") -> (w1302:string)
                    n472 = local read "Calib Path"() -> (w1303:path)
                    n473 = Build Path(base path=w1303, name or relative path=w1302) -> (appended path=w1304:path)
                    n474 = call <vilib>:"Check if File or Folder Exists.vi"("path"=w1304) -> ("file or folder exists?"=w1298:bool, "dup path"=w1299:path)  [unwired: 8 in, 1 out]
                    n475 = case shown="False" w1298 {
                      tunnel: w1299 -> [_ w1313]
                      tunnel: w1297 -> [w1307 _]
                      tunnel: w1296 -> [w1312 _]
                      frame #0 {
                        n476 = Delete From Array(array=w1312, index=w1307) -> (array with subset deleted=w1308:string[])  [unwired: 1 in, 1 out]
                        n477 = Array Size(array=w1308) -> (size(s)=w1311:i32)
                        n478 = Decrement(x=w1311) -> (x-1=w1309:i32)
                        n479 = In Range and Coerce(upper limit=w1309, x=w1307, lower limit=0) -> (coerced(x)=w1306:i32)  [unwired: 1 out]
                        n480 = property on="List of calibrations" class="LstBox (strict)"("Item Names"=w1308, "Val(Sgnl)"=w1306) -> ()  [unwired: 2 in, 2 out]
                      }
                      frame #1 {
                        n481 = stacked-sequence {
                          tunnel: w1313 -> [w1321 _ _]
                          frame #0 {
                            w1314 = 0 ("line index")
                            n482 = Read from Text File(file (use dialog)=w1321) -> (text=w1317:string)  [unwired: 3 in, 3 out]
                            n483 = Spreadsheet String To Array(format string="%e", spreadsheet string=w1317) -> (array=w1319:dbl[][])  [unwired: 2 in]
                            n484 = Pick Line(multi-line string=w1317, line index=w1314) -> (output string=w1316:string)  [unwired: 1 in]
                            n485 = while {
                              shift-right: [w1323] -> _
                              shift-left: w1316 -> [w1326]
                              tunnel: [w1324] -> w1318 mode=indexing
                              stop <- w1322 stop-if-true
                              n486 = Match Pattern(string=w1326, regular expression="\t") -> (before substring=w1324:string, after substring=w1323:string)  [unwired: 1 in, 2 out]
                              n487 = Empty String/Path?(string/path=w1323) -> (empty?=w1322:bool)
                            }
                            n488 = Delete From Array(array=w1319, index (row)=w1314) -> (array with subset deleted=w1315:dbl[][])  [unwired: 2 in, 1 out]
                            n489 = local write "Calibration"(w1315) -> ()
                            n490 = local write "Titles"(w1318) -> ()
                          }
                          frame #1 {
                            n491 = local read "Calibration"() -> (w1331:dbl[][])
                            n492 = call "Sort Calibration.vi"("Calibration (in)"=w1331) -> ("Abs Powers"=w1328:dbl[], "Abs Energies"=w1329:dbl[], "Calibration (out)"=w1330:dbl[][], "Indexes"=w1327:dbl[])  [unwired: 7 in]
                            n493 = local write "Calibration"(w1330) -> ()
                            n494 = local write "Abs Energies"(w1329) -> ()
                            n495 = local write "Abs Powers"(w1328) -> ()
                            n496 = local write "Indexes"(w1327) -> ()
                          }
                          frame #2 {
                            n497 = local read "Manual Mode"() -> (w1332:bool)
                            n498 = case shown="True" w1332 {
                              frame #0 {
                                n499 = local read "Delays (s)"() -> (w1333:dbl[])
                                n500 = property on="Delays (s)" class="Arr (strict)"("Val(Sgnl)"=w1333) -> ()  [unwired: 2 in, 2 out]
                              }
                              frame #1 {
                                n501 = local read "Max. Power (W)"() -> (w1334:dbl)
                                n502 = property on="Max. Power (W)" class="DigNum (strict)"("Val(Sgnl)"=w1334) -> ()  [unwired: 2 in, 2 out]
                              }
                            }
                          }
                        }
                      }
                    }
                  }
                  frame #1 {
                    n503 = stacked-sequence {
                      frame #0 {
                        w1338 = TRUE ("Manual Mode")
                        n504 = local write "Titles"(string[] []) -> ()
                        n505 = local write "Calibration"(dbl[][] []) -> ()
                        n506 = local write "Manual Mode"(w1338) -> ()
                        n507 = local read "Delays (s)"() -> (w1337:dbl[])
                        n508 = Select(t=u8 0, s=w1338, f=u8 2) -> (s? t:f=w1336:u8)
                        n509 = Select(t=u8 2, s=w1338, f=u8 0) -> (s? t:f=w1335:u8)
                        n510 = property on="VISA Box" class="VISAName"("DisabledEnum"=w1336) -> ()  [unwired: 2 in, 2 out]
                        n511 = property on="Delays (s)" class="Arr (strict)"("DisabledEnum"=w1336) -> ()  [unwired: 2 in, 2 out]
                        n512 = property on="Slide Style" class="CmbBox"("DisabledEnum"=w1335) -> ()  [unwired: 2 in, 2 out]
                        n513 = property on="Slide (%,W,J)" class="Slide (strict)"("DisabledEnum"=w1335) -> ()  [unwired: 2 in, 2 out]
                        n514 = property on="Delays (s)" class="Arr (strict)"("Val(Sgnl)"=w1337) -> ()  [unwired: 2 in, 2 out]
                      }
                      frame #1 {
                        n515 = local read "Manual Mode"() -> (w1346:bool)
                        n516 = Select(t=u8 0, s=w1346, f=u8 2) -> (s? t:f=w1345:u8)
                        n517 = property on="Num 4" class="DigNum (strict)"("DisabledEnum"=w1345) -> ()  [unwired: 2 in, 2 out]
                        n518 = property on="Num 5" class="DigNum (strict)"("DisabledEnum"=w1345) -> ()  [unwired: 2 in, 2 out]
                        n519 = property on="Num 6" class="DigNum (strict)"("DisabledEnum"=w1345) -> ()  [unwired: 2 in, 2 out]
                        n520 = property on="Num 7" class="DigNum (strict)"("DisabledEnum"=w1345) -> ()  [unwired: 2 in, 2 out]
                        n521 = property on="Num 8" class="DigNum (strict)"("DisabledEnum"=w1345) -> ()  [unwired: 2 in, 2 out]
                        n522 = property on="Num 9" class="DigNum (strict)"("DisabledEnum"=w1345) -> ()  [unwired: 2 in, 2 out]
                        n523 = property on="Num 10" class="DigNum (strict)"("DisabledEnum"=w1345) -> ()  [unwired: 2 in, 2 out]
                        n524 = property on="Num 11" class="DigNum (strict)"("DisabledEnum"=w1345) -> ()  [unwired: 2 in, 2 out]
                        n525 = property on="Num 12" class="DigNum (strict)"("DisabledEnum"=w1345) -> ()  [unwired: 2 in, 2 out]
                        n526 = property on="Num 13" class="DigNum (strict)"("DisabledEnum"=w1345) -> ()  [unwired: 2 in, 2 out]
                        n527 = property on="Num 14" class="DigNum (strict)"("DisabledEnum"=w1345) -> ()  [unwired: 2 in, 2 out]
                        n528 = property on="Num 15" class="DigNum (strict)"("DisabledEnum"=w1345) -> ()  [unwired: 2 in, 2 out]
                        n529 = property on="Channel" class="CmbBox"("DisabledEnum"=w1345) -> ()  [unwired: 2 in, 2 out]
                        n530 = property on="Num 1" class="DigNum (strict)"("DisabledEnum"=w1345) -> ()  [unwired: 2 in, 2 out]
                        n531 = property on="Num 2" class="DigNum (strict)"("DisabledEnum"=w1345) -> ()  [unwired: 2 in, 2 out]
                        n532 = property on="Num 3" class="DigNum (strict)"("DisabledEnum"=w1345) -> ()  [unwired: 2 in, 2 out]
                      }
                    }
                  }
                }
              }
            }
          }
          event #10 {
            n533 = event-data() -> ()  [unwired: 1 in, 1 out]
            n534 = stacked-sequence {
              frame #0 {
                n535 = local write "Busy"(TRUE ("Busy")) -> ()
                n536 = local read "Heads Numbers"() -> (w1354:i16[])
                n537 = local read "Pulsar Handle"() -> (w1357:i16)
                n538 = local read "OphirFastX"() -> (w1361:refnum<k7>)
                n539 = local read "Heads"() -> (w1355:i32)
                n540 = Index Array(array=w1354, index=w1355) -> (element=w1353:i16)
                n541 = control-ref of="Mode"() -> (w1362:refnum<vi>)
                n542 = call "Set Mode.vi"("Ref Mode"=w1362, "Head Channel"=w1353, "Pulsar Handle"=w1357, "OphirFastX (in)"=w1361) -> ("error out"=w1356:errorcluster, "OphirFastX (out)"=w1358:refnum<k7>)  [unwired: 6 in]
                n543 = call "Save Settings.vi"("error in"=w1356, "Head Channel"=w1353, "Pulsar Handle"=w1357, "OphirFastX (in)"=w1358) -> ("error out"=w1359:errorcluster, "OphirFastX (out)"=w1360:refnum<k7>)  [unwired: 6 in]
                n544 = local write "OphirFastX"(w1360) -> ()
                n545 = local write "Error Setting Head"(w1359) -> ()
              }
              frame #1 {
                n546 = local read "Active Channels"() -> (w1363:T2)
                n547 = local read "Delays (s)"() -> (w1377:dbl[])
                n548 = local read "Mode"() -> (w1375:string)
                n549 = local read "Calibration"() -> (w1378:dbl[][])
                n550 = Match Pattern(string=w1375, regular expression="Power") -> (offset past match=w1373:i32)  [unwired: 1 in, 3 out]
                n551 = call "Simulator.vi"("Proportions"=dbl[] [0.0, 0.0, 0.5, 0.5], "Delays (s)"=w1377, "Active Channels"=w1363, "Calibration"=w1378) -> ("Output Energy (J)"=w1371:dbl, "Output Power (W)"=w1372:dbl)  [unwired: 6 in]
                n552 = Greater Or Equal To 0?(x=w1373) -> (x >= 0?=w1366:bool)
                n553 = Select(t=w1372, s=w1366, f=w1371) -> (s? t:f=w1364:dbl)
                n554 = local read "Abs Energies"() -> (w1369:dbl[])
                n555 = local read "Abs Powers"() -> (w1370:dbl[])
                n556 = Select(t=w1370, s=w1366, f=w1369) -> (s? t:f=w1368:dbl[])
                n557 = local read "Slide Style"() -> (w1367:string)
                n558 = case shown="\"Relative\"" w1367 {
                  tunnel: w1368 -> [_ w1385]
                  tunnel: w1364 -> [w1379 w1381]
                  tunnel: [w1379 w1380] -> w1365
                  frame #0 {
                  }
                  frame #1 {
                    n559 = Array Max & Min(array=w1385) -> (max value=w1384:dbl)  [unwired: 3 out]
                    n560 = Divide(x=w1381, y=w1384) -> (x/y=w1383:dbl)
                    n561 = Multiply(x=w1383, y=100.0) -> (x*y=w1380:dbl)
                  }
                }
                n562 = local write "Slide (%,W,J)"(w1365) -> ()
              }
              frame #2 {
                n563 = local read "Range"() -> (w1400:string)
                n564 = property on="Range" class="CmbBox"("Val(Sgnl)"=w1400) -> ()  [unwired: 2 in, 2 out]
                n565 = local read "Mode"() -> (w1399:string)
                n566 = Match Pattern(string=w1399, regular expression="Power") -> (offset past match=w1397:i32)  [unwired: 1 in, 3 out]
                n567 = Greater Or Equal To 0?(x=w1397) -> (x >= 0?=w1391:bool)
                n568 = Select(t="Power (W)" ("Y Scale.Name Label.Text"), s=w1391, f="Energy (J)" ("Y Scale.Name Label.Text")) -> (s? t:f=w1394:string)
                n569 = Select(t=" (W)" ("Y Scale.Name Label.Text"), s=w1391, f=" (J)" ("Y Scale.Name Label.Text")) -> (s? t:f=w1388:string)
                n570 = property on="Display" class="WFGraph (strict)"("YScale.NameLbl.Text"=w1394) -> ()  [unwired: 2 in, 2 out]
                n571 = property on="Measure" class="DigNum (strict)"("Caption.Text"=w1394) -> ()  [unwired: 2 in, 2 out]
                n572 = Concatenate Strings("Mean" ("string"), w1388) -> (w1387:string)
                n573 = Concatenate Strings("Std. Dev." ("string"), w1388) -> (w1386:string)
                n574 = property on="Average" class="DigNum (strict)"("Caption.Text"=w1387) -> ()  [unwired: 2 in, 2 out]
                n575 = property on="Standard Dev." class="DigNum (strict)"("Caption.Text"=w1386) -> ()  [unwired: 2 in, 2 out]
              }
            }
          }
          event #11 {
            n576 = event-data() -> ()  [unwired: 1 in, 1 out]
            n577 = stacked-sequence {
              frame #0 {
                n578 = local write "Busy"(TRUE ("Busy")) -> ()
                n579 = local read "Heads Numbers"() -> (w1406:i16[])
                n580 = local read "Pulsar Handle"() -> (w1411:i16)
                n581 = local read "OphirFastX"() -> (w1410:refnum<k7>)
                n582 = local read "Heads"() -> (w1407:i32)
                n583 = Index Array(array=w1406, index=w1407) -> (element=w1405:i16)
                n584 = local read "Error Setting Head"() -> (w1409:errorcluster)
                n585 = control-ref of="Range"() -> (w1429:refnum<vi>)
                n586 = call "Set Range.vi"("Ref Range"=w1429, "error in"=w1409, "Head Channel"=w1405, "Pulsar Handle"=w1411, "OphirFastX (in)"=w1410) -> ("error out"=w1427:errorcluster, "OphirFastX (out)"=w1428:refnum<k7>)  [unwired: 5 in]
                n587 = control-ref of="Wavelength (nm)"() -> (w1430:refnum<vi>)
                n588 = call "Set Wavelength.vi"("Ref Wavelength"=w1430, "error in"=w1427, "Head Channel"=w1405, "Pulsar Handle"=w1411, "OphirFastX (in)"=w1428) -> ("error out"=w1423:errorcluster, "OphirFastX (out)"=w1426:refnum<k7>)  [unwired: 5 in]
                n589 = control-ref of="Pulse Length"() -> (w1422:refnum<vi>)
                n590 = call "Set Pulse Length.vi"("Ref Pulse Range"=w1422, "error in"=w1423, "Head Channel"=w1405, "Pulsar Handle"=w1411, "OphirFastX (in)"=w1426) -> ("error out"=w1413:errorcluster, "OphirFastX (out)"=w1415:refnum<k7>)  [unwired: 5 in]
                n591 = control-ref of="Ext. Trigger"() -> (w1408:refnum<vi>)
                n592 = call "Set Ext Trigger On-Off.vi"("Ext. Trigger"=w1408, "error in"=w1413, "Head Channel"=w1405, "Pulsar Handle"=w1411, "OphirFastX (in)"=w1415) -> ("error out"=w1412:errorcluster, "OphirFastX (out)"=w1414:refnum<k7>)  [unwired: 5 in]
                n593 = control-ref of="Trigger Mode"() -> (w1421:refnum<vi>)
                n594 = call "Set Ext Trigger Mode.vi"("Ref Trigger Mode"=w1421, "error in"=w1412, "Pulsar Handle"=w1411, "OphirFastX (in)"=w1414) -> ("error out"=w1418:errorcluster, "OphirFastX (out)"=w1420:refnum<k7>)  [unwired: 6 in]
                n595 = control-ref of="Window Time (us)"() -> (w1416:refnum<vi>)
                n596 = call "Set Window Time.vi"("Ref Window Time"=w1416, "error in"=w1418, "Pulsar Handle"=w1411, "OphirFastX (in)"=w1420) -> ("error out"=w1417:errorcluster, "OphirFastX (out)"=w1419:refnum<k7>)  [unwired: 6 in]
                n597 = call "Save Settings.vi"("error in"=w1417, "Head Channel"=w1405, "Pulsar Handle"=w1411, "OphirFastX (in)"=w1419) -> ("error out"=→"Error Setting Head":errorcluster, "OphirFastX (out)"=w1425:refnum<k7>)  [unwired: 6 in]
                n598 = local write "OphirFastX"(w1425) -> ()
              }
              frame #1 {
                n599 = property on="Range" class="CmbBox"() -> ("Strings[]"=w1432:string[])  [unwired: 2 in, 2 out]
                n600 = for {
                  tunnel: w1432 -> [w1433] mode=indexing
                  tunnel: [w1436] -> w1431 mode=indexing
                  n601 = xnode "Match Regular Expression"("input string"=w1433, "regular expression"="[0-9]{1,4}\\.?[0-9]{0,2}") -> ("whole match"=w1443:string)  [unwired: 4 in, 4 out]
                  n602 = xnode "Match Regular Expression"("input string"=w1433, "regular expression"="m(J|W)") -> ("offset past match"=w1435:i32)  [unwired: 4 in, 4 out]
                  n603 = xnode "Match Regular Expression"("input string"=w1433, "regular expression"="u(J|W)") -> ("offset past match"=w1434:i32)  [unwired: 4 in, 4 out]
                  n604 = Scan Value(string=w1443, format string="%f") -> (value=w1437:dbl)  [unwired: 1 in, 1 out]
                  n605 = Greater Or Equal To 0?(x=w1435) -> (x >= 0?=w1439:bool)
                  n606 = Greater Or Equal To 0?(x=w1434) -> (x >= 0?=w1438:bool)
                  n607 = case shown="False" w1439 {
                    tunnel: w1438 -> [w1661 _]
                    tunnel: w1437 -> [w1660 w1667]
                    tunnel: [w1659 w1666] -> w1436
                    frame #0 {
                      n608 = case shown="False" w1661 {
                        tunnel: w1660 -> [w1662 w1665]
                        tunnel: [w1662 w1663] -> w1659
                        frame #0 {
                        }
                        frame #1 {
                          n609 = Multiply(x=1e-06, y=w1665) -> (x*y=w1663:dbl)
                        }
                      }
                    }
                    frame #1 {
                      n610 = Multiply(x=0.001, y=w1667) -> (x*y=w1666:dbl)
                    }
                  }
                }
                n611 = local write "Range (Numeric)"(w1431) -> ()
              }
              frame #2 {
                n612 = local read "Trigger Mode"() -> (w1782:string)
                n613 = Match Pattern(string=w1782, regular expression="Edge") -> (offset past match=w1784:i32)  [unwired: 1 in, 3 out]
                n614 = local read "Ext. Trigger"() -> (w1777:bool)
                n615 = Greater Or Equal To 0?(x=w1784) -> (x >= 0?=w1776:bool)
                n616 = And(x=w1777, y=w1776) -> (x .and. y?=w1778:bool)
                n617 = Select(t=u8 0, s=w1777, f=u8 2) -> (s? t:f=w1785:u8)
                n618 = Select(t=u8 0, s=w1778, f=u8 2) -> (s? t:f=w1779:u8)
                n619 = property on="Trigger Mode" class="CmbBox"("DisabledEnum"=w1785) -> ()  [unwired: 2 in, 2 out]
                n620 = property on="Window Time (us)" class="DigNum (strict)"("DisabledEnum"=w1779) -> ()  [unwired: 2 in, 2 out]
              }
              frame #3 {
                n621 = local read "Max. Power (W)"() -> (w1788:dbl)
                n622 = property on="Max. Power (W)" class="DigNum (strict)"("Val(Sgnl)"=w1788) -> ()  [unwired: 2 in, 2 out]
              }
            }
          }
          event #12 {
            n623 = event-data() -> ()  [unwired: 1 in, 1 out]
            n624 = stacked-sequence {
              frame #0 {
                n625 = local write "Busy"(TRUE ("Busy")) -> ()
                n626 = local read "Mode"() -> (w1802:string)
                n627 = Match Pattern(string=w1802, regular expression="Power") -> (offset past match=w1800:i32)  [unwired: 1 in, 3 out]
                n628 = Greater Or Equal To 0?(x=w1800) -> (x >= 0?=w1796:bool)
                n629 = local read "Abs Energies"() -> (w1798:dbl[])
                n630 = local read "Abs Powers"() -> (w1799:dbl[])
                n631 = local read "Slide (%,W,J)"() -> (w1794:dbl)
                n632 = Select(t=w1799, s=w1796, f=w1798) -> (s? t:f=w1797:dbl[])
                n633 = local read "Max. Power (W)"() -> (w1792:dbl)
                n634 = local read "Slide Style"() -> (w1795:string)
                n635 = case shown="\"Absolute\"" w1795 {
                  tunnel: w1797 -> [w1806 w1815]
                  tunnel: w1794 -> [w1805 w1811]
                  tunnel: [w1804 w1810] -> w1793
                  frame #0 {
                    n636 = Array Max & Min(array=w1806) -> (max value=w1809:dbl)  [unwired: 3 out]
                    n637 = Multiply(x=w1805, y=w1809) -> (x*y=w1808:dbl)
                    n638 = Divide(x=w1808, y=100.0) -> (x/y=w1804:dbl)
                  }
                  frame #1 {
                    n639 = Array Max & Min(array=w1815) -> (max value=w1814:dbl)  [unwired: 3 out]
                    n640 = Divide(x=w1811, y=w1814) -> (x/y=w1813:dbl)
                    n641 = Multiply(x=w1813, y=100.0) -> (x*y=w1810:dbl)
                  }
                }
                n642 = property on="Max. Power (W)" class="DigNum (strict)"("Val(Sgnl)"=w1792) -> ()  [unwired: 2 in, 2 out]
                n643 = local write "Slide (%,W,J)"(w1793) -> ()
              }
            }
          }
          event #13 {
            n644 = event-data() -> ()  [unwired: 1 in, 1 out]
            n645 = stacked-sequence {
              frame #0 {
                n646 = local write "Busy"(TRUE ("Busy")) -> ()
                n647 = local read "Mode"() -> (w1823:string)
                n648 = Match Pattern(string=w1823, regular expression="Power") -> (offset past match=w1821:i32)  [unwired: 1 in, 3 out]
                n649 = Greater Or Equal To 0?(x=w1821) -> (x >= 0?=w1820:bool)
                n650 = local read "Slide Style"() -> (w1819:string)
                n651 = case shown="\"Relative\", Default" w1819 {
                  tunnel: w1820 -> [w1836 w1844]
                  frame #0 {
                    n652 = local read "Max. Power (W)"() -> (w1827:dbl)
                    n653 = local read "Max. Energy (J)"() -> (w1826:dbl)
                    n654 = Select(t=0.05 ("Data Entry Limits:Increment"), s=w1836, f=0.005 ("Data Entry Limits:Increment")) -> (s? t:f=w1831:dbl)
                    n655 = Select(t=w1827, s=w1836, f=w1826) -> (s? t:f=w1828:dbl)
                    n656 = Select(t="Power (W)" ("Caption.Text"), s=w1836, f="Energy (J)" ("Caption.Text")) -> (s? t:f=w1832:string)
                    n657 = local read "Slide (%,W,J)"() -> (w1825:dbl)
                    n658 = property on="Slide (%,W,J)" class="Slide (strict)"("Val(Sgnl)"=w1825, "Increment"=w1831, "Maximum"=w1828, "Scale.Maximum"=w1828, "Minimum"=0.0 ("Data Entry Limits:Minimum"), "Caption.Text"=w1832) -> ()  [unwired: 2 in, 2 out]
                  }
                  frame #1 {
                    w1838 = 100.0 ("Data Entry Limits:Maximum")
                    n659 = Select(t="Power (%)" ("Caption.Text"), s=w1844, f="Energy (%)" ("Caption.Text")) -> (s? t:f=w1839:string)
                    n660 = local read "Slide (%,W,J)"() -> (w1837:dbl)
                    n661 = property on="Slide (%,W,J)" class="Slide (strict)"("Val(Sgnl)"=w1837, "Increment"=0.5 ("Data Entry Limits:Increment"), "Maximum"=w1838, "Scale.Maximum"=w1838, "Minimum"=0.0 ("Data Entry Limits:Minimum"), "Caption.Text"=w1839) -> ()  [unwired: 2 in, 2 out]
                  }
                }
              }
            }
          }
          event #14 {
            n662 = event-data() -> ()  [unwired: 1 in, 1 out]
            n663 = stacked-sequence {
              frame #0 {
                w1849 = 1000000000000.0 ("y")
                n664 = local read "Mode"() -> (w1859:string)
                n665 = local write "Busy"(TRUE ("Busy")) -> ()
                n666 = Match Pattern(string=w1859, regular expression="Power") -> (offset past match=w1857:i32)  [unwired: 1 in, 3 out]
                n667 = Greater Or Equal To 0?(x=w1857) -> (x >= 0?=w1856:bool)
                n668 = local read "Abs Energies"() -> (w1854:dbl[])
                n669 = local read "Abs Powers"() -> (w1855:dbl[])
                n670 = Select(t=w1855, s=w1856, f=w1854) -> (s? t:f=w1853:dbl[])
                n671 = local read "Slide (%,W,J)"() -> (w1865:dbl)
                n672 = local read "Slide Style"() -> (w1866:string)
                n673 = case shown="\"Relative\", Default" w1866 {
                  tunnel: [w1870 w1875] -> w1862
                  tunnel: w1865 -> [w1874 w1875]
                  tunnel: w1853 -> [w1869 _]
                  frame #0 {
                    n674 = Divide(x=w1874, y=100.0) -> (x/y=w1872:dbl)
                    n675 = Array Max & Min(array=w1869) -> (max value=w1871:dbl)  [unwired: 3 out]
                    n676 = Multiply(x=w1871, y=w1872) -> (x*y=w1870:dbl)
                  }
                  frame #1 {
                  }
                }
                n677 = local read "Indexes"() -> (w1863:dbl[])
                n678 = Threshold 1D Array(2:w1862, 3:w1853) -> (0:w1861:dbl)  [unwired: 1 in]
                n679 = local read "Calibration"() -> (w1864:dbl[][])
                n680 = Transpose 2D Array(2D array=w1864) -> (transposed array=w1868:dbl[][])
                n681 = for {
                  N: 4 -> [_]
                  tunnel: w1868 -> [w1882] mode=indexing
                  tunnel: w1863 -> [w1881]
                  tunnel: w1861 -> [w1880]
                  tunnel: [w1876] -> w1852 mode=indexing
                  n682 = Build Array(w1880) -> (w1879:dbl[])
                  n683 = call <vilib>:"Interpolate 1D.vi"("X is monotonic"=TRUE, "xi"=w1879, "X"=w1881, "Y"=w1882) -> ("yi"=w1877:dbl[])  [unwired: 5 in, 2 out]
                  n684 = Index Array(array=w1877) -> (element=w1876:dbl)  [unwired: 1 in]
                }
                n685 = Multiply(x=w1852, y=w1849) -> (x*y=w1851:dbl[])
                n686 = Round To Nearest(number=w1851) -> (nearest integer value=w1850:dbl[])
                n687 = Divide(x=w1850, y=w1849) -> (x/y=w1848:dbl[])
                n688 = property on="Delays (s)" class="Arr (strict)"("Val(Sgnl)"=w1848) -> ()  [unwired: 2 in, 2 out]
              }
            }
          }
          event #15 {
            n689 = event-data() -> ()  [unwired: 1 in, 1 out]
            n690 = stacked-sequence {
              frame #0 {
                n691 = local write "Busy"(TRUE ("Busy")) -> ()
                n692 = for {
                  N: 15 -> [_]
                  i -> [w1888]
                  n693 = case shown="0, Default" w1888 {
                    frame #0 {
                      n694 = local read "Num 15"() -> (w1890:i32)
                      n695 = local read "Num 14"() -> (w1889:i32)
                      n696 = Less Than 0?(x=w1890) -> (x < 0?=w1893:bool)
                      n697 = case shown="False" w1893 {
                        tunnel: w1890 -> [w1895 _]
                        tunnel: [w1899 9 ("Num 2")] -> w1892
                        tunnel: [w1898 w1907] -> w1891
                        tunnel: w1890 -> [w1897 _]
                        tunnel: w1889 -> [w1894 w1906]
                        frame #0 {
                          n698 = Equal?(x=10 ("y"), y=w1895) -> (x = y?=w1900:bool)
                          n699 = case shown="True" w1900 {
                            tunnel: [0 ("Num 2") w1905] -> w1899
                            tunnel: [w1902 w1904] -> w1898
                            tunnel: w1897 -> [_ w1905]
                            tunnel: w1894 -> [w1901 w1904]
                            frame #0 {
                              n700 = Increment(x=w1901) -> (x+1=w1902:i32)
                            }
                            frame #1 {
                            }
                          }
                        }
                        frame #1 {
                          n701 = Decrement(x=w1906) -> (x-1=w1907:i32)
                        }
                      }
                      n702 = local write "Num 15"(w1892) -> ()
                      n703 = local write "Num 14"(w1891) -> ()
                    }
                    frame #1 {
                      n704 = local read "Num 14"() -> (w1910:i32)
                      n705 = local read "Num 13"() -> (w1909:i32)
                      n706 = Less Than 0?(x=w1910) -> (x < 0?=w1913:bool)
                      n707 = case shown="False" w1913 {
                        tunnel: w1910 -> [w1915 _]
                        tunnel: [w1919 9 ("Num 2")] -> w1912
                        tunnel: [w1918 w1927] -> w1911
                        tunnel: w1910 -> [w1917 _]
                        tunnel: w1909 -> [w1914 w1926]
                        frame #0 {
                          n708 = Equal?(x=10 ("y"), y=w1915) -> (x = y?=w1920:bool)
                          n709 = case shown="False" w1920 {
                            tunnel: [0 ("Num 2") w1925] -> w1919
                            tunnel: [w1922 w1924] -> w1918
                            tunnel: w1917 -> [_ w1925]
                            tunnel: w1914 -> [w1921 w1924]
                            frame #0 {
                              n710 = Increment(x=w1921) -> (x+1=w1922:i32)
                            }
                            frame #1 {
                            }
                          }
                        }
                        frame #1 {
                          n711 = Decrement(x=w1926) -> (x-1=w1927:i32)
                        }
                      }
                      n712 = local write "Num 14"(w1912) -> ()
                      n713 = local write "Num 13"(w1911) -> ()
                    }
                    frame #2 {
                      n714 = local read "Num 13"() -> (w1930:i32)
                      n715 = local read "Num 12"() -> (w1929:i32)
                      n716 = Less Than 0?(x=w1930) -> (x < 0?=w1933:bool)
                      n717 = case shown="True" w1933 {
                        tunnel: w1930 -> [w1935 _]
                        tunnel: [w1939 9 ("Num 2")] -> w1932
                        tunnel: [w1938 w1947] -> w1931
                        tunnel: w1930 -> [w1937 _]
                        tunnel: w1929 -> [w1934 w1946]
                        frame #0 {
                          n718 = Equal?(x=10 ("y"), y=w1935) -> (x = y?=w1940:bool)
                          n719 = case shown="False" w1940 {
                            tunnel: [0 ("Num 2") w1945] -> w1939
                            tunnel: [w1942 w1944] -> w1938
                            tunnel: w1937 -> [_ w1945]
                            tunnel: w1934 -> [w1941 w1944]
                            frame #0 {
                              n720 = Increment(x=w1941) -> (x+1=w1942:i32)
                            }
                            frame #1 {
                            }
                          }
                        }
                        frame #1 {
                          n721 = Decrement(x=w1946) -> (x-1=w1947:i32)
                        }
                      }
                      n722 = local write "Num 13"(w1932) -> ()
                      n723 = local write "Num 12"(w1931) -> ()
                    }
                    frame #3 {
                      n724 = local read "Num 12"() -> (w1950:i32)
                      n725 = local read "Num 11"() -> (w1949:i32)
                      n726 = Less Than 0?(x=w1950) -> (x < 0?=w1953:bool)
                      n727 = case shown="False" w1953 {
                        tunnel: w1950 -> [w1955 _]
                        tunnel: [w1959 9 ("Num 2")] -> w1952
                        tunnel: [w1958 w1967] -> w1951
                        tunnel: w1950 -> [w1957 _]
                        tunnel: w1949 -> [w1954 w1966]
                        frame #0 {
                          n728 = Equal?(x=10 ("y"), y=w1955) -> (x = y?=w1960:bool)
                          n729 = case shown="False" w1960 {
                            tunnel: [0 ("Num 2") w1965] -> w1959
                            tunnel: [w1962 w1964] -> w1958
                            tunnel: w1957 -> [_ w1965]
                            tunnel: w1954 -> [w1961 w1964]
                            frame #0 {
                              n730 = Increment(x=w1961) -> (x+1=w1962:i32)
                            }
                            frame #1 {
                            }
                          }
                        }
                        frame #1 {
                          n731 = Decrement(x=w1966) -> (x-1=w1967:i32)
                        }
                      }
                      n732 = local write "Num 12"(w1952) -> ()
                      n733 = local write "Num 11"(w1951) -> ()
                    }
                    frame #4 {
                      n734 = local read "Num 11"() -> (w1970:i32)
                      n735 = local read "Num 10"() -> (w1969:i32)
                      n736 = Less Than 0?(x=w1970) -> (x < 0?=w1973:bool)
                      n737 = case shown="False" w1973 {
                        tunnel: w1970 -> [w1975 _]
                        tunnel: [w1979 9 ("Num 2")] -> w1972
                        tunnel: [w1978 w1987] -> w1971
                        tunnel: w1970 -> [w1977 _]
                        tunnel: w1969 -> [w1974 w1986]
                        frame #0 {
                          n738 = Equal?(x=10 ("y"), y=w1975) -> (x = y?=w1980:bool)
                          n739 = case shown="False" w1980 {
                            tunnel: [0 ("Num 2") w1985] -> w1979
                            tunnel: [w1982 w1984] -> w1978
                            tunnel: w1977 -> [_ w1985]
                            tunnel: w1974 -> [w1981 w1984]
                            frame #0 {
                              n740 = Increment(x=w1981) -> (x+1=w1982:i32)
                            }
                            frame #1 {
                            }
                          }
                        }
                        frame #1 {
                          n741 = Decrement(x=w1986) -> (x-1=w1987:i32)
                        }
                      }
                      n742 = local write "Num 11"(w1972) -> ()
                      n743 = local write "Num 10"(w1971) -> ()
                    }
                    frame #5 {
                      n744 = local read "Num 10"() -> (w1990:i32)
                      n745 = local read "Num 9"() -> (w1989:i32)
                      n746 = Less Than 0?(x=w1990) -> (x < 0?=w1993:bool)
                      n747 = case shown="False" w1993 {
                        tunnel: w1990 -> [w1995 _]
                        tunnel: [w1999 9 ("Num 2")] -> w1992
                        tunnel: [w1998 w2007] -> w1991
                        tunnel: w1990 -> [w1997 _]
                        tunnel: w1989 -> [w1994 w2006]
                        frame #0 {
                          n748 = Equal?(x=10 ("y"), y=w1995) -> (x = y?=w2000:bool)
                          n749 = case shown="False" w2000 {
                            tunnel: [0 ("Num 2") w2005] -> w1999
                            tunnel: [w2002 w2004] -> w1998
                            tunnel: w1997 -> [_ w2005]
                            tunnel: w1994 -> [w2001 w2004]
                            frame #0 {
                              n750 = Increment(x=w2001) -> (x+1=w2002:i32)
                            }
                            frame #1 {
                            }
                          }
                        }
                        frame #1 {
                          n751 = Decrement(x=w2006) -> (x-1=w2007:i32)
                        }
                      }
                      n752 = local write "Num 10"(w1992) -> ()
                      n753 = local write "Num 9"(w1991) -> ()
                    }
                    frame #6 {
                      n754 = local read "Num 9"() -> (w2010:i32)
                      n755 = local read "Num 8"() -> (w2009:i32)
                      n756 = Less Than 0?(x=w2010) -> (x < 0?=w2013:bool)
                      n757 = case shown="False" w2013 {
                        tunnel: w2010 -> [w2015 _]
                        tunnel: [w2019 9 ("Num 2")] -> w2012
                        tunnel: [w2018 w2027] -> w2011
                        tunnel: w2010 -> [w2017 _]
                        tunnel: w2009 -> [w2014 w2026]
                        frame #0 {
                          n758 = Equal?(x=10 ("y"), y=w2015) -> (x = y?=w2020:bool)
                          n759 = case shown="False" w2020 {
                            tunnel: [0 ("Num 2") w2025] -> w2019
                            tunnel: [w2022 w2024] -> w2018
                            tunnel: w2017 -> [_ w2025]
                            tunnel: w2014 -> [w2021 w2024]
                            frame #0 {
                              n760 = Increment(x=w2021) -> (x+1=w2022:i32)
                            }
                            frame #1 {
                            }
                          }
                        }
                        frame #1 {
                          n761 = Decrement(x=w2026) -> (x-1=w2027:i32)
                        }
                      }
                      n762 = local write "Num 9"(w2012) -> ()
                      n763 = local write "Num 8"(w2011) -> ()
                    }
                    frame #7 {
                      n764 = local read "Num 8"() -> (w2030:i32)
                      n765 = local read "Num 7"() -> (w2029:i32)
                      n766 = Less Than 0?(x=w2030) -> (x < 0?=w2033:bool)
                      n767 = case shown="False" w2033 {
                        tunnel: w2030 -> [w2035 _]
                        tunnel: [w2039 9 ("Num 2")] -> w2032
                        tunnel: [w2038 w2047] -> w2031
                        tunnel: w2030 -> [w2037 _]
                        tunnel: w2029 -> [w2034 w2046]
                        frame #0 {
                          n768 = Equal?(x=10 ("y"), y=w2035) -> (x = y?=w2040:bool)
                          n769 = case shown="False" w2040 {
                            tunnel: [0 ("Num 2") w2045] -> w2039
                            tunnel: [w2042 w2044] -> w2038
                            tunnel: w2037 -> [_ w2045]
                            tunnel: w2034 -> [w2041 w2044]
                            frame #0 {
                              n770 = Increment(x=w2041) -> (x+1=w2042:i32)
                            }
                            frame #1 {
                            }
                          }
                        }
                        frame #1 {
                          n771 = Decrement(x=w2046) -> (x-1=w2047:i32)
                        }
                      }
                      n772 = local write "Num 8"(w2032) -> ()
                      n773 = local write "Num 7"(w2031) -> ()
                    }
                    frame #8 {
                      n774 = local read "Num 7"() -> (w2050:i32)
                      n775 = local read "Num 6"() -> (w2049:i32)
                      n776 = Less Than 0?(x=w2050) -> (x < 0?=w2053:bool)
                      n777 = case shown="False" w2053 {
                        tunnel: w2050 -> [w2055 _]
                        tunnel: [w2059 9 ("Num 2")] -> w2052
                        tunnel: [w2058 w2067] -> w2051
                        tunnel: w2050 -> [w2057 _]
                        tunnel: w2049 -> [w2054 w2066]
                        frame #0 {
                          n778 = Equal?(x=10 ("y"), y=w2055) -> (x = y?=w2060:bool)
                          n779 = case shown="False" w2060 {
                            tunnel: [0 ("Num 2") w2065] -> w2059
                            tunnel: [w2062 w2064] -> w2058
                            tunnel: w2057 -> [_ w2065]
                            tunnel: w2054 -> [w2061 w2064]
                            frame #0 {
                              n780 = Increment(x=w2061) -> (x+1=w2062:i32)
                            }
                            frame #1 {
                            }
                          }
                        }
                        frame #1 {
                          n781 = Decrement(x=w2066) -> (x-1=w2067:i32)
                        }
                      }
                      n782 = local write "Num 7"(w2052) -> ()
                      n783 = local write "Num 6"(w2051) -> ()
                    }
                    frame #9 {
                      n784 = local read "Num 6"() -> (w2070:i32)
                      n785 = local read "Num 5"() -> (w2069:i32)
                      n786 = Less Than 0?(x=w2070) -> (x < 0?=w2073:bool)
                      n787 = case shown="False" w2073 {
                        tunnel: w2070 -> [w2075 _]
                        tunnel: [w2079 9 ("Num 2")] -> w2072
                        tunnel: [w2078 w2087] -> w2071
                        tunnel: w2070 -> [w2077 _]
                        tunnel: w2069 -> [w2074 w2086]
                        frame #0 {
                          n788 = Equal?(x=10 ("y"), y=w2075) -> (x = y?=w2080:bool)
                          n789 = case shown="False" w2080 {
                            tunnel: [0 ("Num 2") w2085] -> w2079
                            tunnel: [w2082 w2084] -> w2078
                            tunnel: w2077 -> [_ w2085]
                            tunnel: w2074 -> [w2081 w2084]
                            frame #0 {
                              n790 = Increment(x=w2081) -> (x+1=w2082:i32)
                            }
                            frame #1 {
                            }
                          }
                        }
                        frame #1 {
                          n791 = Decrement(x=w2086) -> (x-1=w2087:i32)
                        }
                      }
                      n792 = local write "Num 6"(w2072) -> ()
                      n793 = local write "Num 5"(w2071) -> ()
                    }
                    frame #10 {
                      n794 = local read "Num 5"() -> (w2090:i32)
                      n795 = local read "Num 4"() -> (w2089:i32)
                      n796 = Less Than 0?(x=w2090) -> (x < 0?=w2093:bool)
                      n797 = case shown="False" w2093 {
                        tunnel: w2090 -> [w2095 _]
                        tunnel: [w2099 9 ("Num 2")] -> w2092
                        tunnel: [w2098 w2107] -> w2091
                        tunnel: w2090 -> [w2097 _]
                        tunnel: w2089 -> [w2094 w2106]
                        frame #0 {
                          n798 = Equal?(x=10 ("y"), y=w2095) -> (x = y?=w2100:bool)
                          n799 = case shown="False" w2100 {
                            tunnel: [0 ("Num 2") w2105] -> w2099
                            tunnel: [w2102 w2104] -> w2098
                            tunnel: w2097 -> [_ w2105]
                            tunnel: w2094 -> [w2101 w2104]
                            frame #0 {
                              n800 = Increment(x=w2101) -> (x+1=w2102:i32)
                            }
                            frame #1 {
                            }
                          }
                        }
                        frame #1 {
                          n801 = Decrement(x=w2106) -> (x-1=w2107:i32)
                        }
                      }
                      n802 = local write "Num 5"(w2092) -> ()
                      n803 = local write "Num 4"(w2091) -> ()
                    }
                    frame #11 {
                      n804 = local read "Num 4"() -> (w2110:i32)
                      n805 = local read "Num 3"() -> (w2109:i32)
                      n806 = Less Than 0?(x=w2110) -> (x < 0?=w2113:bool)
                      n807 = case shown="False" w2113 {
                        tunnel: w2110 -> [w2115 _]
                        tunnel: [w2119 9 ("Num 2")] -> w2112
                        tunnel: [w2118 w2127] -> w2111
                        tunnel: w2110 -> [w2117 _]
                        tunnel: w2109 -> [w2114 w2126]
                        frame #0 {
                          n808 = Equal?(x=10 ("y"), y=w2115) -> (x = y?=w2120:bool)
                          n809 = case shown="False" w2120 {
                            tunnel: [0 ("Num 2") w2125] -> w2119
                            tunnel: [w2122 w2124] -> w2118
                            tunnel: w2117 -> [_ w2125]
                            tunnel: w2114 -> [w2121 w2124]
                            frame #0 {
                              n810 = Increment(x=w2121) -> (x+1=w2122:i32)
                            }
                            frame #1 {
                            }
                          }
                        }
                        frame #1 {
                          n811 = Decrement(x=w2126) -> (x-1=w2127:i32)
                        }
                      }
                      n812 = local write "Num 4"(w2112) -> ()
                      n813 = local write "Num 3"(w2111) -> ()
                    }
                    frame #12 {
                      n814 = local read "Num 3"() -> (w2130:i32)
                      n815 = local read "Num 2"() -> (w2129:i32)
                      n816 = Less Than 0?(x=w2130) -> (x < 0?=w2133:bool)
                      n817 = case shown="False" w2133 {
                        tunnel: w2130 -> [w2135 _]
                        tunnel: [w2139 9 ("Num 2")] -> w2132
                        tunnel: [w2138 w2147] -> w2131
                        tunnel: w2130 -> [w2137 _]
                        tunnel: w2129 -> [w2134 w2146]
                        frame #0 {
                          n818 = Equal?(x=10 ("y"), y=w2135) -> (x = y?=w2140:bool)
                          n819 = case shown="False" w2140 {
                            tunnel: [0 ("Num 2") w2145] -> w2139
                            tunnel: [w2142 w2144] -> w2138
                            tunnel: w2137 -> [_ w2145]
                            tunnel: w2134 -> [w2141 w2144]
                            frame #0 {
                              n820 = Increment(x=w2141) -> (x+1=w2142:i32)
                            }
                            frame #1 {
                            }
                          }
                        }
                        frame #1 {
                          n821 = Decrement(x=w2146) -> (x-1=w2147:i32)
                        }
                      }
                      n822 = local write "Num 3"(w2132) -> ()
                      n823 = local write "Num 2"(w2131) -> ()
                    }
                    frame #13 {
                      n824 = local read "Num 2"() -> (w2150:i32)
                      n825 = local read "Num 1"() -> (w2149:i32)
                      n826 = Less Than 0?(x=w2150) -> (x < 0?=w2153:bool)
                      n827 = case shown="False" w2153 {
                        tunnel: w2150 -> [w2155 _]
                        tunnel: [w2159 9 ("Num 2")] -> w2152
                        tunnel: [w2158 w2167] -> w2151
                        tunnel: w2150 -> [w2157 _]
                        tunnel: w2149 -> [w2154 w2166]
                        frame #0 {
                          n828 = Equal?(x=10 ("y"), y=w2155) -> (x = y?=w2160:bool)
                          n829 = case shown="True" w2160 {
                            tunnel: [0 ("Num 2") w2165] -> w2159
                            tunnel: [w2162 w2164] -> w2158
                            tunnel: w2157 -> [_ w2165]
                            tunnel: w2154 -> [w2161 w2164]
                            frame #0 {
                              n830 = Increment(x=w2161) -> (x+1=w2162:i32)
                            }
                            frame #1 {
                            }
                          }
                        }
                        frame #1 {
                          n831 = Decrement(x=w2166) -> (x-1=w2167:i32)
                        }
                      }
                      n832 = local write "Num 2"(w2152) -> ()
                      n833 = local write "Num 1"(w2151) -> ()
                    }
                    frame #14 {
                      n834 = local read "Num 1"() -> (w2169:i32)
                      n835 = Less Than 0?(x=w2169) -> (x < 0?=w2171:bool)
                      n836 = case shown="False" w2171 {
                        tunnel: w2169 -> [w2172 _]
                        tunnel: [w2175 0 ("Num 2")] -> w2170
                        tunnel: w2169 -> [w2174 _]
                        frame #0 {
                          n837 = Equal?(x=10 ("y"), y=w2172) -> (x = y?=w2176:bool)
                          n838 = case shown="False" w2176 {
                            tunnel: [9 ("Num 2") w2178] -> w2175
                            tunnel: w2174 -> [_ w2178]
                            frame #0 {
                            }
                            frame #1 {
                            }
                          }
                        }
                        frame #1 {
                        }
                      }
                      n839 = local write "Num 1"(w2170) -> ()
                    }
                  }
                }
              }
              frame #1 {
                w2180 = 3 ("length (rest)")
                n840 = for {
                  N: 15 -> [_]
                  shift-right: [w2198] -> w2185
                  shift-left: "" -> [w2199]
                  i -> [w2202]
                  n841 = case shown="0, Default" w2202 {
                    tunnel: [w2203 w2204 w2205 w2206 w2207 w2208 w2209 w2210 w2211 w2212 w2213 w2214 w2215 w2216 w2217] -> w2201
                    frame #0 {
                      n842 = local read "Num 1"() -> (w2203:i32)
                    }
                    frame #1 {
                      n843 = local read "Num 2"() -> (w2204:i32)
                    }
                    frame #2 {
                      n844 = local read "Num 3"() -> (w2205:i32)
                    }
                    frame #3 {
                      n845 = local read "Num 4"() -> (w2206:i32)
                    }
                    frame #4 {
                      n846 = local read "Num 5"() -> (w2207:i32)
                    }
                    frame #5 {
                      n847 = local read "Num 6"() -> (w2208:i32)
                    }
                    frame #6 {
                      n848 = local read "Num 7"() -> (w2209:i32)
                    }
                    frame #7 {
                      n849 = local read "Num 8"() -> (w2210:i32)
                    }
                    frame #8 {
                      n850 = local read "Num 9"() -> (w2211:i32)
                    }
                    frame #9 {
                      n851 = local read "Num 10"() -> (w2212:i32)
                    }
                    frame #10 {
                      n852 = local read "Num 11"() -> (w2213:i32)
                    }
                    frame #11 {
                      n853 = local read "Num 12"() -> (w2214:i32)
                    }
                    frame #12 {
                      n854 = local read "Num 13"() -> (w2215:i32)
                    }
                    frame #13 {
                      n855 = local read "Num 14"() -> (w2216:i32)
                    }
                    frame #14 {
                      n856 = local read "Num 15"() -> (w2217:i32)
                    }
                  }
                  n857 = Number To Decimal String(number=w2201) -> (decimal integer string=w2200:string)  [unwired: 1 in]
                  n858 = Concatenate Strings(w2199, w2200) -> (w2198:string)
                }
                n859 = String Subset(string=w2185, length (rest)=w2180) -> (substring=w2183:string)  [unwired: 1 in]
                n860 = String Subset(string=w2185, offset (0)=w2180) -> (substring=w2182:string)  [unwired: 1 in]
                n861 = local read "Channel"() -> (w2192:string)
                n862 = case shown="\"C\"" w2192 {
                  tunnel: [0 1 2 3] -> w2188
                  frame #0 {
                  }
                  frame #1 {
                  }
                  frame #2 {
                  }
                  frame #3 {
                  }
                }
                n863 = Concatenate Strings(w2183, "." ("string"), w2182) -> (w2181:string)
                n864 = Scan Value(string=w2181, format string="%g") -> (value=w2190:dbl)  [unwired: 1 in, 1 out]
                n865 = local read "Delays (s)"() -> (w2189:dbl[])
                n866 = Replace Array Subset(array=w2189, new element=w2190, index=w2188) -> (w2187:dbl[])
                n867 = property on="Delays (s)" class="Arr (strict)"("Val(Sgnl)"=w2187) -> ()  [unwired: 2 in, 2 out]
              }
            }
          }
          event #16 {
            n868 = event-data() -> ()  [unwired: 1 in, 1 out]
            n869 = stacked-sequence {
              frame #0 {
                n870 = local write "Busy"(TRUE ("Busy")) -> ()
                n871 = local read "VISA Box"() -> (w2221:refnum<visa-resource-name>)
                n872 = First Call?() -> (First Call?: T/F=w2227:bool)
                n873 = case shown="True" w2227 {
                  tunnel: w2221 -> [w2229 w2237]
                  tunnel: [w2232 w2234] -> w2226
                  tunnel: [w2231 w2235] -> w2225
                  tunnel: [errorcluster {"status"=FALSE, "code"=0, "source"=""} ("Error Writing") w2236] -> w2224
                  tunnel: [w2229 w2233] -> w2222
                  frame #0 {
                    n874 = local read "Modes"() -> (w2231:cluster{"A=":u16, "B=":u16, "C=":u16, "D=":u16})
                    n875 = local read "Delays (s)"() -> (w2232:dbl[])
                  }
                  frame #1 {
                    n876 = stacked-sequence {
                      tunnel: w2237 -> [w2246 _]
                      tunnel: [w2243 _] -> w2236
                      tunnel: [_ w2247] -> w2235
                      tunnel: [_ w2248] -> w2234
                      tunnel: [w2240 _] -> w2233
                      frame #0 {
                        n877 = property class="Instr"(reference=w2246) -> (reference out=w2240:refnum<visa-resource-name>, "Primary Addr"=w2238:u16)  [unwired: 1 in, 1 out]
                        n878 = Number To Decimal String(number=w2238) -> (decimal integer string=w2245:string)  [unwired: 1 in]
                        n879 = call "Read Box.vi"("GPIB Address"=w2245) -> ("Error Reading"=→"Error Reading Delay Box":errorcluster, "Reading"=w2244:string[], "Error Writing"=w2243:errorcluster)  [unwired: 6 in]
                        n880 = call "Apply Box.vi"("Reading"=w2244) -> ("Modes"=w2242:cluster{"A=":u16, "B=":u16, "C=":u16, "D=":u16}, "Delays (s)"=w2241:dbl[])  [unwired: 3 in]
                        n881 = local write "Modes"(w2242) -> ()
                        n882 = local write "Delays (s)"(w2241) -> ()
                      }
                      frame #1 {
                        n883 = local read "Delays (s)"() -> (w2249:dbl[])
                        n884 = local read "Modes"() -> (w2250:cluster{"A=":u16, "B=":u16, "C=":u16, "D=":u16})
                        n885 = call "Confirm Delays.vi"("Modes"=w2250, "Delays (s)"=w2249) -> ("Modes (out)"=w2247:cluster{"A=":u16, "B=":u16, "C=":u16, "D=":u16}, "Delays (s) (out)"=w2248:dbl[])  [unwired: 2 in]
                        n886 = local write "Delays (s)"(w2248) -> ()
                        n887 = local write "Modes"(w2247) -> ()
                      }
                    }
                  }
                }
                n888 = call "dg535 delay.vi"("Delays (A,B,C,D)"=w2226, "VISA resource name"=w2222, "Modes"=w2225, "error in"=w2224) -> ("error out"=→"Error Writing Delay Box":errorcluster)  [unwired: 5 in]
              }
              frame #1 {
                w2252 = i16 15 ("width (-)")
                n889 = local read "Channel"() -> (w2258:string)
                n890 = case shown="\"A\", Default" w2258 {
                  tunnel: [0 1 2 3] -> w2257
                  frame #0 {
                  }
                  frame #1 {
                  }
                  frame #2 {
                  }
                  frame #3 {
                  }
                }
                n891 = local read "Delays (s)"() -> (w2256:dbl[])
                n892 = Index Array(array=w2256, index=w2257) -> (element=w2251:dbl)
                n893 = Multiply(x=1000000000000.0, y=w2251) -> (x*y=w2254:dbl)
                n894 = Number To Decimal String(number=w2254, width (-)=w2252) -> (decimal integer string=w2253:string)
                n895 = for {
                  N: w2252 -> [_]
                  tunnel: w2253 -> [w2263]
                  i -> [w2260]
                  n896 = String Subset(string=w2263, offset (0)=w2260, length (rest)=1 ("length (rest)")) -> (substring=w2261:string)
                  n897 = Decimal String To Number(string=w2261) -> (number=w2259:i32)  [unwired: 2 in, 1 out]
                  n898 = case shown="0, Default" w2260 {
                    tunnel: w2259 -> [w2264 w2265 w2266 w2267 w2268 w2269 w2270 w2271 w2272 w2273 w2274 w2275 w2276 w2277 w2278]
                    frame #0 {
                      n899 = local write "Num 1"(w2264) -> ()
                    }
                    frame #1 {
                      n900 = local write "Num 2"(w2265) -> ()
                    }
                    frame #2 {
                      n901 = local write "Num 3"(w2266) -> ()
                    }
                    frame #3 {
                      n902 = local write "Num 4"(w2267) -> ()
                    }
                    frame #4 {
                      n903 = local write "Num 5"(w2268) -> ()
                    }
                    frame #5 {
                      n904 = local write "Num 6"(w2269) -> ()
                    }
                    frame #6 {
                      n905 = local write "Num 7"(w2270) -> ()
                    }
                    frame #7 {
                      n906 = local write "Num 8"(w2271) -> ()
                    }
                    frame #8 {
                      n907 = local write "Num 9"(w2272) -> ()
                    }
                    frame #9 {
                      n908 = local write "Num 10"(w2273) -> ()
                    }
                    frame #10 {
                      n909 = local write "Num 11"(w2274) -> ()
                    }
                    frame #11 {
                      n910 = local write "Num 12"(w2275) -> ()
                    }
                    frame #12 {
                      n911 = local write "Num 13"(w2276) -> ()
                    }
                    frame #13 {
                      n912 = local write "Num 14"(w2277) -> ()
                    }
                    frame #14 {
                      n913 = local write "Num 15"(w2278) -> ()
                    }
                  }
                }
              }
            }
          }
          event #17 {
            n914 = event-data() -> ()  [unwired: 1 in, 1 out]
            n915 = local write "Busy"(TRUE ("Busy")) -> ()
            n916 = stacked-sequence {
              frame #0 {
                n917 = local read "VISA Box"() -> (w2287:refnum<visa-resource-name>)
                n918 = property class="Instr"(reference=w2287) -> ("Primary Addr"=w2294:u16)  [unwired: 1 in, 2 out]
                n919 = Number To Decimal String(number=w2294) -> (decimal integer string=w2293:string)  [unwired: 1 in]
                n920 = call "Read Box.vi"("GPIB Address"=w2293) -> ("Error Reading"=w2289:errorcluster, "Reading"=w2292:string[], "Error Writing"=w2288:errorcluster)  [unwired: 6 in]
                n921 = local write "Error Writing Delay Box"(w2288) -> ()
                n922 = call "Apply Box.vi"("Reading"=w2292) -> ("Modes"=w2291:cluster{"A=":u16, "B=":u16, "C=":u16, "D=":u16}, "Delays (s)"=w2290:dbl[])  [unwired: 3 in]
                n923 = local write "Error Reading Delay Box"(w2289) -> ()
                n924 = local write "Modes"(w2291) -> ()
                n925 = local write "Delays (s)"(w2290) -> ()
              }
              frame #1 {
                n926 = local read "Delays (s)"() -> (w2297:dbl[])
                n927 = local read "Modes"() -> (w2298:cluster{"A=":u16, "B=":u16, "C=":u16, "D=":u16})
                n928 = call "Confirm Delays.vi"("Modes"=w2298, "Delays (s)"=w2297) -> ("Modes (out)"=w2296:cluster{"A=":u16, "B=":u16, "C=":u16, "D=":u16}, "Delays (s) (out)"=w2295:dbl[])  [unwired: 2 in]
                n929 = property on="Delays (s)" class="Arr (strict)"("Val(Sgnl)"=w2295) -> ()  [unwired: 2 in, 2 out]
                n930 = local write "Modes"(w2296) -> ()
              }
            }
          }
        }
      }
      frame #1 {
        n931 = stacked-sequence {
          tunnel: [_ _ _ _ w2485 _ _ _ _ _ _ _ _] -> w2302
          tunnel: [_ _ _ _ _ _ _ _ _ _ _ w2928 _] -> w2301
          tunnel: [_ _ _ _ _ w2498 _ _ _ _ _ _ _] -> w2300
          tunnel: w2299 -> [_ _ _ _ _ _ _ _ _ _ _ _ _]
          frame #0 {
            n932 = control-ref of="This VI"() -> (w2313:refnum<vi>)
            n933 = property class="VI"(reference=w2313) -> (reference out=w2305:refnum<vi>, "Path"=w2310:path)  [unwired: 1 in, 1 out]
            n934 = Path To String(path=w2310) -> (string=w2309:string)
            n935 = xnode "Match Regular Expression"("input string"=w2309, "regular expression"="(\\\\|\\/|:)(pecon|Controller)\\..+$") -> ("before match"=w2308:string)  [unwired: 4 in, 4 out]
            n936 = call "ConfigFile Name.vi"() -> ("ConfigFile Name"=w2312:string)  [unwired: 5 in]
            n937 = String To Path(string=w2308) -> (path=w2307:path)
            n938 = Build Path(base path=w2307, name or relative path=w2312) -> (appended path=w2306:path)
            n939 = call <vilib>:"Check if File or Folder Exists.vi"("path"=w2306) -> ("file or folder exists?"=w2314:bool, "dup path"=w2315:path)  [unwired: 8 in, 1 out]
            n940 = case shown="True" w2314 {
              tunnel: w2305 -> [_ w2424]
              tunnel: w2315 -> [_ w2423]
              frame #0 {
              }
              frame #1 {
                n941 = call "Config File Reader (VI Ref).vi"("This VI"=w2424, "Config File Path"=w2423) -> ()  [unwired: 9 in, 1 out]
              }
            }
          }
          frame #1 {
            w2431 = TRUE ("Manual Mode")
            n942 = local write "Manual Mode"(w2431) -> ()
            n943 = local read "Autoscale"() -> (w2427:bool)
            n944 = Select(t=u8 0, s=w2431, f=u8 2) -> (s? t:f=w2426:u8)
            n945 = Select(t=u8 2, s=w2431, f=u8 0) -> (s? t:f=w2425:u8)
            n946 = Select(t=u8 2, s=w2427, f=u8 0) -> (s? t:f=w2430:u8)
            n947 = property on="Range" class="CmbBox"("DisabledEnum"=w2430) -> ()  [unwired: 2 in, 2 out]
            n948 = property on="VISA Box" class="VISAName"("DisabledEnum"=w2426) -> ()  [unwired: 2 in, 2 out]
            n949 = property on="Delays (s)" class="Arr (strict)"("DisabledEnum"=w2426) -> ()  [unwired: 2 in, 2 out]
            n950 = property on="Slide Style" class="CmbBox"("DisabledEnum"=w2425) -> ()  [unwired: 2 in, 2 out]
            n951 = property on="Slide (%,W,J)" class="Slide (strict)"("DisabledEnum"=w2425) -> ()  [unwired: 2 in, 2 out]
          }
          frame #2 {
            n952 = local read "Manual Mode"() -> (w2437:bool)
            n953 = Select(t=u8 0, s=w2437, f=u8 2) -> (s? t:f=w2436:u8)
            n954 = property on="Num 4" class="DigNum (strict)"("DisabledEnum"=w2436) -> ()  [unwired: 2 in, 2 out]
            n955 = property on="Num 5" class="DigNum (strict)"("DisabledEnum"=w2436) -> ()  [unwired: 2 in, 2 out]
            n956 = property on="Num 6" class="DigNum (strict)"("DisabledEnum"=w2436) -> ()  [unwired: 2 in, 2 out]
            n957 = property on="Num 7" class="DigNum (strict)"("DisabledEnum"=w2436) -> ()  [unwired: 2 in, 2 out]
            n958 = property on="Num 8" class="DigNum (strict)"("DisabledEnum"=w2436) -> ()  [unwired: 2 in, 2 out]
            n959 = property on="Num 9" class="DigNum (strict)"("DisabledEnum"=w2436) -> ()  [unwired: 2 in, 2 out]
            n960 = property on="Num 10" class="DigNum (strict)"("DisabledEnum"=w2436) -> ()  [unwired: 2 in, 2 out]
            n961 = property on="Num 11" class="DigNum (strict)"("DisabledEnum"=w2436) -> ()  [unwired: 2 in, 2 out]
            n962 = property on="Num 12" class="DigNum (strict)"("DisabledEnum"=w2436) -> ()  [unwired: 2 in, 2 out]
            n963 = property on="Num 13" class="DigNum (strict)"("DisabledEnum"=w2436) -> ()  [unwired: 2 in, 2 out]
            n964 = property on="Num 14" class="DigNum (strict)"("DisabledEnum"=w2436) -> ()  [unwired: 2 in, 2 out]
            n965 = property on="Num 15" class="DigNum (strict)"("DisabledEnum"=w2436) -> ()  [unwired: 2 in, 2 out]
            n966 = property on="Channel" class="CmbBox"("DisabledEnum"=w2436) -> ()  [unwired: 2 in, 2 out]
            n967 = property on="Num 1" class="DigNum (strict)"("DisabledEnum"=w2436) -> ()  [unwired: 2 in, 2 out]
            n968 = property on="Num 2" class="DigNum (strict)"("DisabledEnum"=w2436) -> ()  [unwired: 2 in, 2 out]
            n969 = property on="Num 3" class="DigNum (strict)"("DisabledEnum"=w2436) -> ()  [unwired: 2 in, 2 out]
          }
          frame #3 {
            n970 = local read "OphirFastX"() -> (w2455:refnum<k7>)
            n971 = call "Initialize USB.vi"("OphirFastX (in)"=w2455) -> ("error out"=w2456:errorcluster, "OphirFastX (out)"=w2457:refnum<k7>)  [unwired: 9 in]
            n972 = call "Get Pulsar Info.vi"("error in"=w2456, "OphirFastX (in)"=w2457) -> ("error out"=w2458:errorcluster, "Pulsar Handle"=w2453:i16, "OphirFastX (out)"=w2459:refnum<k7>, "Device Found?"=w2454:bool, "Pulsar Info"=w2446:string)  [unwired: 5 in]
            n973 = local write "Pulsar Info"(w2446) -> ()
            n974 = local write "Found?"(w2454) -> ()
            n975 = local write "Pulsar Handle"(w2453) -> ()
            n976 = call "Get Number of Channels.vi"("Pulsar Info"=w2446) -> ("# Channels"=w2447:i32)  [unwired: 4 in]
            n977 = for {
              N: w2447 -> [_]
              tunnel: w2453 -> [w2472]
              shift-right: [w2471] -> w2450
              shift-left: w2458 -> [w2473]
              shift-right: [w2470] -> w2451
              shift-left: w2459 -> [w2474]
              shift-right: [w2463] -> w2444
              shift-left: string[] [] -> [w2464]
              shift-right: [w2460] -> w2449
              shift-left: i32[] [] -> [w2461]
              i -> [w2462]
              n978 = call <vilib>:"Space Constant.vi"() -> ("String"=w2469:string)
              n979 = Concatenate Strings(w2469, w2469, "0" ("string")) -> (w2466:string)
              n980 = call "Get Head Info.vi"("error in"=w2473, "Head Channel"=w2462, "Pulsar Handle"=w2472, "OphirFastX (in)"=w2474) -> ("error out"=w2471:errorcluster, "OphirFastX (out)"=w2470:refnum<k7>, "Head Info"=w2465:string)  [unwired: 5 in]
              n981 = Not Equal?(x=w2465, y=w2466) -> (x != y?=w2467:bool)
              n982 = case shown="True" w2467 {
                tunnel: w2465 -> [_ w2482]
                tunnel: w2464 -> [w2476 w2481]
                tunnel: [w2476 w2480] -> w2463
                tunnel: w2462 -> [_ w2479]
                tunnel: w2461 -> [w2475 w2478]
                tunnel: [w2475 w2477] -> w2460
                frame #0 {
                }
                frame #1 {
                  n983 = Build Array (concatenate)(w2478, w2479) -> (w2477:i32[])
                  n984 = Build Array (concatenate)(w2481, w2482) -> (w2480:string[])
                }
              }
            }
            n985 = local write "Heads Numbers"(w2449) -> ()
            n986 = local write "OphirFastX"(w2451) -> ()
            n987 = local write "Error Initializing Head"(w2450) -> ()
            n988 = Array Size(array=w2444) -> (size(s)=w2445:i32)
            n989 = local read "Heads"() -> (w2440:i32)
            n990 = Decrement(x=w2445) -> (x-1=w2442:i32)
            n991 = In Range and Coerce(upper limit=w2442, x=w2440, lower limit=0) -> (coerced(x)=w2443:i32)  [unwired: 1 out]
            n992 = property on="Heads" class="LstBox (strict)"("Item Names"=w2444, "Value"=w2443) -> ()  [unwired: 2 in, 2 out]
          }
          frame #4 {
            n993 = local read "Heads Numbers"() -> (w2483:i16[])
            n994 = local read "Pulsar Handle"() -> (w2487:i16)
            n995 = local read "OphirFastX"() -> (w2484:refnum<k7>)
            n996 = for {
              tunnel: w2487 -> [w2494]
              shift-right: [w2493] -> w2486
              shift-left: w2484 -> [w2492]
              tunnel: w2483 -> [w2491] mode=indexing
              n997 = invoke class="OphirFastX" method="EnableDisableChannelForCS"(reference=w2492, "nDeviceHandle"=w2494, "nHeadChannel"=w2491, "nEnable"=i16 1) -> (reference out=w2496:refnum<k7>, "nDeviceHandle"=w2497:i16)  [unwired: 2 in, 4 out]
              n998 = invoke class="OphirFastX" method="StartCS2"(reference=w2496, "nDeviceHandle"=w2497) -> (reference out=w2493:refnum<k7>)  [unwired: 2 in, 3 out]
            }
            n999 = To Variant(anything="") -> (Variant=w2490:variant)
            n1000 = vi-ref "DataReady Event Callback.vi"() -> ("vi reference"=w2488:refnum<vi>)
            n1001 = Obtain Notifier(notification data type=w2490) -> (notifier out=w2485:refnum<notifier>)  [unwired: 3 in, 2 out]
            n1002 = node(w2484, w2488, w2485) -> ()  [unwired: 2 in, 2 out]
            n1003 = local write "OphirFastX"(w2486) -> ()
          }
          frame #5 {
            n1004 = local read "Min. Size (# Points)"() -> (w2499:i32)
            n1005 = local read "Check Lower Level"() -> (w2505:bool)
            n1006 = local read "Max. Power (W)"() -> (w2503:dbl)
            n1007 = local read "Active Channels"() -> (w2504:T2)
            n1008 = local read "Max. Energy (J)"() -> (w2502:dbl)
            n1009 = local read "Simulate Values"() -> (w2509:bool)
            n1010 = local read "Slide (%,W,J)"() -> (w2501:dbl)
            n1011 = local read "Buffer (units)"() -> (w2508:string)
            n1012 = local read "Manual Mode"() -> (w2514:bool)
            n1013 = local read "Buffer (size)"() -> (w2507:u32)
            n1014 = local read "Ext. Trigger"() -> (w2517:bool)
            n1015 = local read "Graph style"() -> (w2500:string)
            n1016 = local read "Slide Style"() -> (w2511:string)
            n1017 = local read "Delays (s)"() -> (w2513:dbl[])
            n1018 = local read "Calib Path"() -> (w2510:path)
            n1019 = local read "Autoscale"() -> (w2516:bool)
            n1020 = local read "VISA Box"() -> (w2515:refnum<visa-resource-name>)
            n1021 = local read "Acquire"() -> (w2512:bool)
            n1022 = local read "Modes"() -> (w2506:cluster{"A=":u16, "B=":u16, "C=":u16, "D=":u16})
            n1023 = Bundle("Ext. Trigger"=w2517, "Autoscale"=w2516, "Check Lower Level"=w2505, "VISA Box"=w2515, "Manual Mode"=w2514, "Delays (s)"=w2513, "Modes"=w2506, "Active Channels"=w2504, "Graph style"=w2500, "Buffer (size)"=w2507, "Buffer (units)"=w2508, "Min. Size (# Points)"=w2499, "Simulate Values"=w2509, "Calib Path"=w2510, "Slide Style"=w2511, "Max. Power (W)"=w2503, "Max. Energy (J)"=w2502, "Slide (%,W,J)"=w2501, "Acquire"=w2512) -> (w2520:T3)  [unwired: 1 in]
            n1024 = local read "Heads Numbers"() -> (w2519:i16[])
            n1025 = Array Size(array=w2519) -> (size(s)=w2518:i32)
            n1026 = Initialize Array(w2520, w2518) -> (w2498:T4)
          }
          frame #6 {
            n1027 = local read "Error Initializing Head"() -> (w2528:errorcluster)
            n1028 = local read "Heads Numbers"() -> (w2526:i16[])
            n1029 = property on="Heads" class="LstBox (strict)"() -> ("Item Names"=w2527:string[], "Value"=w2525:i32)  [unwired: 2 in, 2 out]
            n1030 = local read "OphirFastX"() -> (w2523:refnum<k7>)
            n1031 = Index Array(array=w2526, index=w2525) -> (element=w2522:i16)
            n1032 = Index Array(array=w2527, index=w2525) -> (element=w2524:string)
            n1033 = local read "Pulsar Handle"() -> (w2521:i16)
            n1034 = control-ref of="Mode"() -> (w2546:refnum<vi>)
            n1035 = local read "Found?"() -> (w2549:bool)
            n1036 = call "Get Mode.vi"("Ref Mode"=w2546, "Device Found?"=w2549, "Head Info"=w2524, "error in"=w2528, "Head Channel"=w2522, "Pulsar Handle"=w2521, "OphirFastX (in)"=w2523) -> ("error out"=w2551:errorcluster, "OphirFastX (out)"=w2550:refnum<k7>)  [unwired: 3 in]
            n1037 = control-ref of="Range"() -> (w2545:refnum<vi>)
            n1038 = call "Get Range.vi"("Ref Range"=w2545, "error in"=w2551, "Head Channel"=w2522, "Pulsar Handle"=w2521, "OphirFastX (in)"=w2550) -> ("error out"=w2548:errorcluster, "OphirFastX (out)"=w2547:refnum<k7>)  [unwired: 5 in]
            n1039 = control-ref of="Wavelength (nm)"() -> (w2544:refnum<vi>)
            n1040 = call "Get Wavelength.vi"("Ref Wavelength"=w2544, "error in"=w2548, "Head Channel"=w2522, "Pulsar Handle"=w2521, "OphirFastX (in)"=w2547) -> ("error out"=w2542:errorcluster, "OphirFastX (out)"=w2543:refnum<k7>)  [unwired: 5 in]
            n1041 = control-ref of="Pulse Length"() -> (w2541:refnum<vi>)
            n1042 = call "Get Pulse Length.vi"("Ref Pulse Length"=w2541, "error in"=w2542, "Head Channel"=w2522, "Pulsar Handle"=w2521, "OphirFastX (in)"=w2543) -> ("error out"=w2539:errorcluster, "OphirFastX (out)"=w2540:refnum<k7>)  [unwired: 5 in]
            n1043 = control-ref of="Ext. Trigger"() -> (w2529:refnum<vi>)
            n1044 = call "Set Ext Trigger On-Off.vi"("Ext. Trigger"=w2529, "error in"=w2539, "Head Channel"=w2522, "Pulsar Handle"=w2521, "OphirFastX (in)"=w2540) -> ("error out"=w2537:errorcluster, "OphirFastX (out)"=w2538:refnum<k7>)  [unwired: 5 in]
            n1045 = control-ref of="Trigger Mode"() -> (w2536:refnum<vi>)
            n1046 = call "Get Ext Trigger Mode.vi"("Ref Trigger Mode"=w2536, "error in"=w2537, "Pulsar Handle"=w2521, "OphirFastX (in)"=w2538) -> ("error out"=w2535:errorcluster, "OphirFastX (out)"=w2531:refnum<k7>)  [unwired: 6 in]
            n1047 = control-ref of="Window Time (us)"() -> (w2532:refnum<vi>)
            n1048 = call "Set Window Time.vi"("Ref Window Time"=w2532, "Pulsar Handle"=w2521, "OphirFastX (in)"=w2531) -> ("OphirFastX (out)"=w2530:refnum<k7>)  [unwired: 7 in, 1 out]
            n1049 = call "Save Settings.vi"("error in"=w2535, "Head Channel"=w2522, "Pulsar Handle"=w2521, "OphirFastX (in)"=w2530) -> ("error out"=→"Error Initializing Head":errorcluster, "OphirFastX (out)"=w2534:refnum<k7>)  [unwired: 6 in]
            n1050 = local write "OphirFastX"(w2534) -> ()
          }
          frame #7 {
            n1051 = property on="Range" class="CmbBox"() -> ("Strings[]"=w2553:string[])  [unwired: 2 in, 2 out]
            n1052 = for {
              tunnel: w2553 -> [w2554] mode=indexing
              tunnel: [w2557] -> w2552 mode=indexing
              n1053 = xnode "Match Regular Expression"("input string"=w2554, "regular expression"="[0-9]{1,4}\\.?[0-9]{0,2}") -> ("whole match"=w2564:string)  [unwired: 4 in, 4 out]
              n1054 = xnode "Match Regular Expression"("input string"=w2554, "regular expression"="m(J|W)") -> ("offset past match"=w2556:i32)  [unwired: 4 in, 4 out]
              n1055 = xnode "Match Regular Expression"("input string"=w2554, "regular expression"="u(J|W)") -> ("offset past match"=w2555:i32)  [unwired: 4 in, 4 out]
              n1056 = Scan Value(string=w2564, format string="%f") -> (value=w2558:dbl)  [unwired: 1 in, 1 out]
              n1057 = Greater Or Equal To 0?(x=w2556) -> (x >= 0?=w2560:bool)
              n1058 = Greater Or Equal To 0?(x=w2555) -> (x >= 0?=w2559:bool)
              n1059 = case shown="False" w2560 {
                tunnel: w2559 -> [w2782 _]
                tunnel: w2558 -> [w2781 w2788]
                tunnel: [w2780 w2787] -> w2557
                frame #0 {
                  n1060 = case shown="True" w2782 {
                    tunnel: w2781 -> [w2783 w2786]
                    tunnel: [w2783 w2784] -> w2780
                    frame #0 {
                    }
                    frame #1 {
                      n1061 = Multiply(x=1e-06, y=w2786) -> (x*y=w2784:dbl)
                    }
                  }
                }
                frame #1 {
                  n1062 = Multiply(x=0.001, y=w2788) -> (x*y=w2787:dbl)
                }
              }
            }
            n1063 = local write "Range (Numeric)"(w2552) -> ()
          }
          frame #8 {
            n1064 = local read "Trigger Mode"() -> (w2903:string)
            n1065 = Match Pattern(string=w2903, regular expression="Edge") -> (offset past match=w2905:i32)  [unwired: 1 in, 3 out]
            n1066 = local read "Ext. Trigger"() -> (w2898:bool)
            n1067 = Greater Or Equal To 0?(x=w2905) -> (x >= 0?=w2897:bool)
            n1068 = And(x=w2898, y=w2897) -> (x .and. y?=w2899:bool)
            n1069 = Select(t=u8 0, s=w2898, f=u8 2) -> (s? t:f=w2906:u8)
            n1070 = Select(t=u8 0, s=w2899, f=u8 2) -> (s? t:f=w2900:u8)
            n1071 = property on="Trigger Mode" class="CmbBox"("DisabledEnum"=w2906) -> ()  [unwired: 2 in, 2 out]
            n1072 = property on="Window Time (us)" class="DigNum (strict)"("DisabledEnum"=w2900) -> ()  [unwired: 2 in, 2 out]
          }
          frame #9 {
            n1073 = local read "Mode"() -> (w2922:string)
            n1074 = Match Pattern(string=w2922, regular expression="Power") -> (offset past match=w2920:i32)  [unwired: 1 in, 3 out]
            n1075 = Greater Or Equal To 0?(x=w2920) -> (x >= 0?=w2914:bool)
            n1076 = Select(t="Power (W)" ("Y Scale.Name Label.Text"), s=w2914, f="Energy (J)" ("Y Scale.Name Label.Text")) -> (s? t:f=w2917:string)
            n1077 = Select(t=" (W)" ("Y Scale.Name Label.Text"), s=w2914, f=" (J)" ("Y Scale.Name Label.Text")) -> (s? t:f=w2911:string)
            n1078 = property on="Display" class="WFGraph (strict)"("YScale.NameLbl.Text"=w2917) -> ()  [unwired: 2 in, 2 out]
            n1079 = property on="Measure" class="DigNum (strict)"("Caption.Text"=w2917) -> ()  [unwired: 2 in, 2 out]
            n1080 = Concatenate Strings("Mean" ("string"), w2911) -> (w2910:string)
            n1081 = Concatenate Strings("Std. Dev." ("string"), w2911) -> (w2909:string)
            n1082 = property on="Average" class="DigNum (strict)"("Caption.Text"=w2910) -> ()  [unwired: 2 in, 2 out]
            n1083 = property on="Standard Dev." class="DigNum (strict)"("Caption.Text"=w2909) -> ()  [unwired: 2 in, 2 out]
          }
          frame #10 {
            n1084 = local read "Heads Numbers"() -> (w2925:i16[])
            n1085 = Array Size(array=w2925) -> (size(s)=w2926:i32)
            n1086 = local read "Min. Size (# Points)"() -> (w2924:i32)
            n1087 = local write "Check Lower Level"(FALSE ("Check Lower Level")) -> ()
            n1088 = Initialize Array(w2924, w2926) -> (w2923:i32[])
            n1089 = local write "Sub-buffer Sizes"(w2923) -> ()
          }
          frame #11 {
            w2939 = u32[] []  # Times (sub-buffer)
            w2938 = dbl[] []  # Graph (sub-buffer)
            w2937 = u32[] []  # Times (main buffer)
            w2936 = dbl[] []  # Graph (main buffer)
            n1090 = local read "Heads Numbers"() -> (w2934:i16[])
            n1091 = Bundle("Graph (main buffer)"=w2936, "Times (main buffer)"=w2937, "Graph (sub-buffer)"=w2938, "Times (sub-buffer)"=w2939) -> (w2935:T5)  [unwired: 1 in]
            n1092 = Array Size(array=w2934) -> (size(s)=w2933:i32)
            n1093 = Initialize Array(w2935, w2933) -> (w2928:T6)
            n1094 = local read "Heads Numbers"() -> (w2931:i16[])
            n1095 = Tick Count (ms)() -> (millisecond timer value=w2930:u32)
            n1096 = Array Size(array=w2931) -> (size(s)=w2932:i32)
            n1097 = Initialize Array(w2930, w2932) -> (w2929:u32[])
            n1098 = local write "T0 (s)"(w2929) -> ()
          }
          frame #12 {
            n1099 = local read "Calib Path"() -> (w2945:path)
            n1100 = List Folder(path=w2945) -> (filenames=w2944:string[], error out=w2948:errorcluster)  [unwired: 3 in, 2 out]
            n1101 = local write "Error Loading Dialog"(w2948) -> ()
            n1102 = for {
              tunnel: w2944 -> [w2951] mode=indexing
              shift-right: [w2954] -> w2941
              shift-left: string[] [] -> [w2955]
              tunnel: ".*[0-9]{4}_[0-9]{4}.*\\.txt" ("pattern") -> [w2953]
              n1103 = xnode "Match Regular Expression"("input string"=w2951, "regular expression"=w2953) -> ("offset past match"=w2956:i32)  [unwired: 4 in, 4 out]
              n1104 = Less Than 0?(x=w2956) -> (x < 0?=w2950:bool)
              n1105 = Match Pattern(string=w2951, regular expression="\\.txt") -> (before substring=w2949:string)  [unwired: 1 in, 3 out]
              n1106 = case shown="False" w2950 {
                tunnel: w2949 -> [w2959 _]
                tunnel: w2955 -> [w2958 w2960]
                tunnel: [w2957 w2960] -> w2954
                frame #0 {
                  n1107 = Build Array (concatenate)(w2958, w2959) -> (w2957:string[])
                }
                frame #1 {
                }
              }
            }
            n1108 = Empty Array?(array=w2941) -> (empty?=w2947:bool)
            n1109 = case shown="False" w2947 {
              tunnel: w2941 -> [w3070 _]
              tunnel: [w3068 -1 ("lower limit")] -> w2946
              frame #0 {
                n1110 = Array Size(array=w3070) -> (size(s)=w3071:i32)
                n1111 = local read "List of calibrations"() -> (w3069:i32)
                n1112 = Decrement(x=w3071) -> (x-1=w3073:i32)
                n1113 = In Range and Coerce(upper limit=w3073, x=w3069, lower limit=0) -> (coerced(x)=w3068:i32)  [unwired: 1 out]
              }
              frame #1 {
              }
            }
            n1114 = call "Sort name chrono.vi"("Names"=w2941) -> ("Names Sorted"=w2940:string[])  [unwired: 4 in]
            n1115 = property on="List of calibrations" class="LstBox (strict)"("Item Names"=w2940, "Val(Sgnl)"=w2946) -> ()  [unwired: 2 in, 2 out]
          }
        }
        n1116 = local write "Busy"(TRUE ("Busy")) -> ()
      }
    }
    "Busy" <- FALSE ("Busy")
  }
